vi "Main_量測.vi"(10 "連線測試":bool) -> ()   [LabVIEW 2015]
uses:
  Setting/0.Control/Setting_Control_Pattern Paremeter.ctl
  <vilib>/vision/Measure.llb/Edge Polarity.ctl
  Setting/0.Control/Setting_Control_Line Paremeter.ctl
  <vilib>/userdefined/High Color/IMAQdx.ctl
  <vilib>/Utility/miscctls.llb/LVPointTypeDef.ctl
  Function/1.0 IO/Control/Main_IO #.ctl
  <vilib>/vision/NI_Vision_Development_Module.lvlib
panel:
  out "狀態： 2":T1
  out "群組： 2":T2
  out "狀態：":string
  out "群組：":string
  out "帳號：":string
  in  "刀數 2":u16
  in  "功率右 2":i32=70 max=80
  in  "掃描速率(刀速)右 2":i32=220 max=2000 format="%0.0f"
  in  "角度(右) 3":dbl min=0.0 max=360.0
  in  "功率左 2":i32=70 max=80
  in  "掃描速率(刀速) 左 2":i32=220 max=2000 format="%0.0f"
  in  "角度(左) 3":dbl min=0.0 max=360.0
  in  "刀數":u16
  in  "功率右":i32=70 max=80
  in  "掃描速率(刀速)右":i32=220 max=2000 format="%0.0f"
  in  "角度(右)":dbl min=0.0 max=360.0
  in  "功率左":i32=70 max=80
  in  "掃描速率(刀速) 左":i32=220 max=2000 format="%0.0f"
  in  "角度(左)":dbl min=0.0 max=360.0
  in  "儲存圖片":bool
  in  "Tab Control":enum32{"影像1", "影像2"}(tab)
  out "Image1":T3(plugin-control)
  in  "pixel轉mm(左)":dbl
  out "總值左out":dbl
  in  "左邊線段":enum16{"加", "減"}(ring)
  in  "左進點":dbl
  in  "影像1左確認":bool
  in  "影像1右確認":bool
  out "總值右out":dbl
  in  "右邊線段":enum16{"加", "減"}(ring)
  in  "右進點":dbl
  out "Image 2":T3(plugin-control)
  in  "pixel轉mm(右)":dbl
  in  "影像2左確認":bool
  out "總值左out 2":dbl
  in  "左進點 2":dbl
  in  "左邊線段 2":enum16{"加", "減"}(ring)
  out "總值右out 2":dbl
  in  "右邊線段 2":enum16{"加", "減"}(ring)
  in  "右進點 2":dbl
  in  "影像2右確認":bool
  in  "代刚":bool
  in  "Enum":enum16{"オ", "右"}(ring)
  in  "代刚":bool
  out "Patttern_R":T3(plugin-control)
  out "Patttern_L":T3(plugin-control)
  out "連線測試 Action":T4
  # "不要的，試機時要拿掉"
  # "mm"
  # "mm"
  # "mm"
  # "mm"
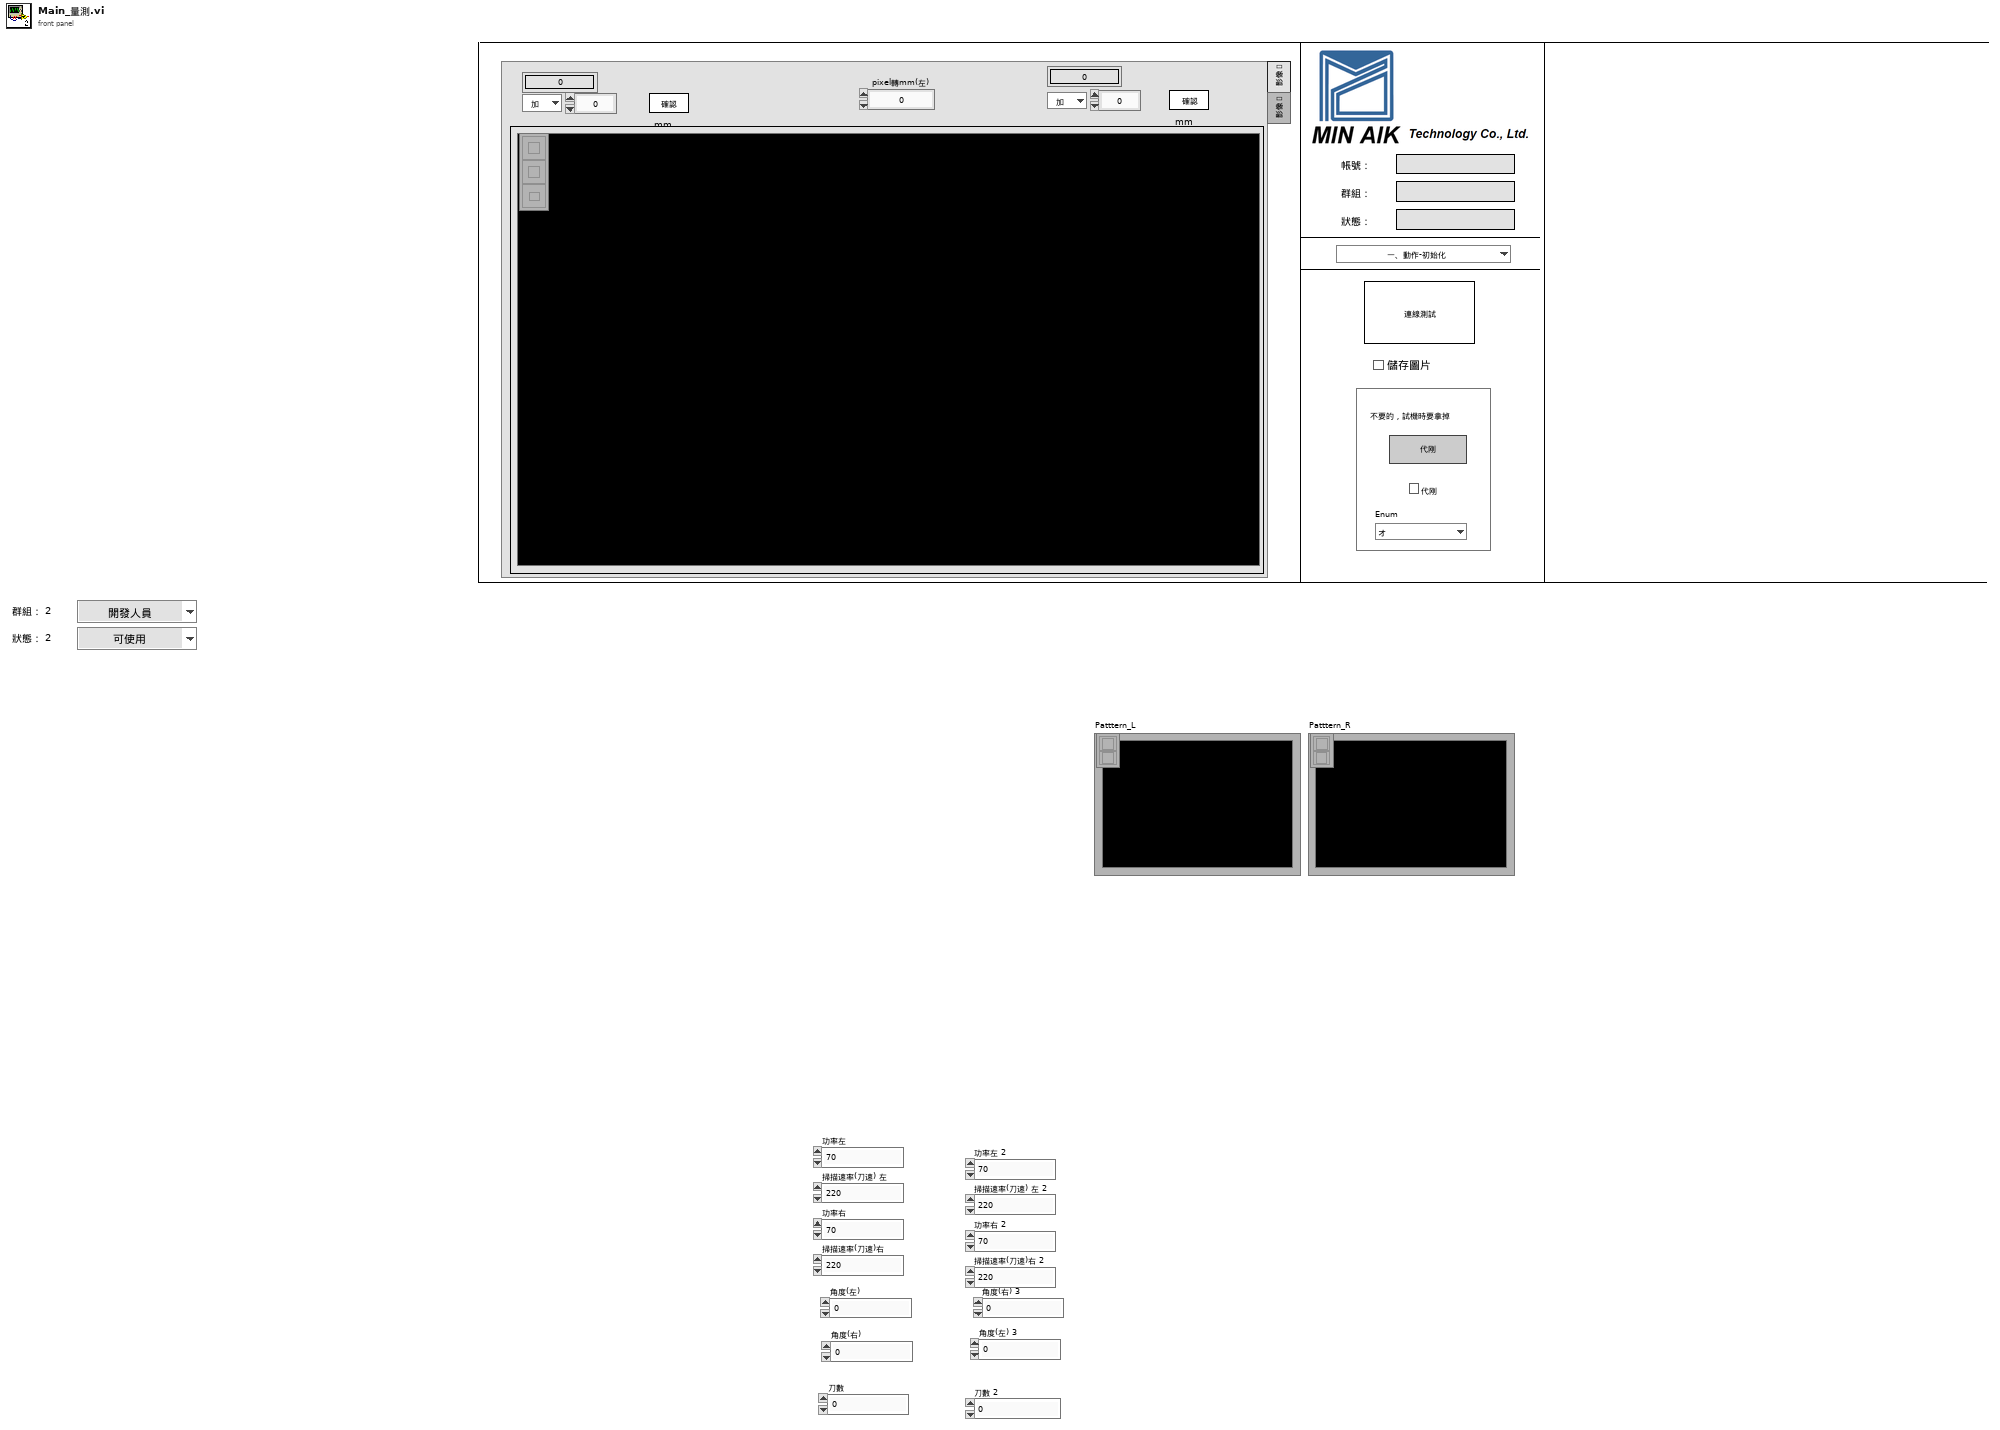
[diagram p1: front panel]
types:
  T1 = typedef "Control_User Accounts_Status.ctl" = enum16{"可使用", "不可使用"}
  T2 = typedef "Control_User account_Permissions.ctl" = enum16{"開發人員", "管理者", "工程師", "作業員"}
  T3 = typedef "IMAQ Image.ctl" = refnum<image>
  T4 = typedef "連線測試_Control_Main Action.ctl" = enum16{"一、動作-初始化", "二、動作-連線測試", "三、動作-離開", "1.0 功能-IO控制", "       1.1 IO-初始化", "       1.2 Set Point(EOT On)第一拍照", "       1.3Set Point(EOT Off)第一拍照", "       1.4Get Point(SOT)第一拍照", "       1.5Set Point(EOT On)第二拍照", "       1.6Set Point(EOT Off)第二拍照", "       1.7Get Point(SOT)第二拍照", "       1.8Set Point(EOT On)第一雷射", "       1.9Set Point(EOT Off)第一雷射", "       1.10Get Point(SOT)第一雷射", "       1.11Set Point(EOT On)第二雷射", "       1.12Set Point(EOT Off)第二雷射", "       1.13Get Point(SOT)第二雷射", "2.0功能-相機控制", "       2.1相機-初始化", "       2.2相機-取像1", "       2.2相機-取像2", "       2.3相機-關閉", "3.0功能-影像控制", "       3.1影像-初始化", "       3.2影像-更新影像", "       3.3影像-儲存影像1", "       3.3影像-儲存影像2", "4.0功能-檢測", "       4.1檢測-初始化", "      4.2浪代-浪代1", "      4.2浪代-浪代2", "      4.3檢測-量測1", "      4.3檢測-量測2", "5.0功能-雷射控制", "      5.1雷射-初始化", "      5.2雷射-寫入數值1", "      5.2雷射-寫入數值2", "      5.3雷射-寫入刀數", "      5.4雷射-讀出數值", "      5.5雷射-切換", "      5.6雷射-雷射觸發", "      5.7雷射-關閉", "6.0功能-檔案", "       6.1檔案-初始化", "       6.2檔案-儲存檔案", "       6.3檔案-開啟檔案(setting)", "       6.3檔案-開啟檔案(點檢)", "       6.3檔案-開啟檔案(近點)", "       6.4檔案-匯入檔案(近點)", "       6.4檔案-開啟檔案(雷射)", "7.0 錯誤", "8.0等待", "       8.1等待(計算時間)", "9.0離開", "10.0功能-機台驗證", "      10.1機台驗證-初始化", "      10.2機台驗證-檢測", "11.0對話視窗"}
  T5 = typedef "Control_Main_All Data.ctl" = enum16{"Initialize", "Set Data", "Get Data"}
  T6 = typedef "LVPointTypeDef.ctl" = cluster{"Horizontal":i16, "Vertical":i16}
  T7 = typedef "Control_User account_Data.ctl" = cluster{"帳號 :":string, "權限等級：":T2, "建立時間：":string, "修改時間：":string, "到期時間：":string, "狀態：":T1, "期限：":T8, "密碼：":string}
  T8 = typedef "Control_User account_Date.ctl" = enum16{"零天", "一天", "七天", "一個月", "一年", "三年"}
  T9 = enum8{"Enabled", "Disabled", "Disabled and Grayed Out"}
  T10 = typedef "IMAQdx.ctl" = refnum<k21>
  T11 = enum16{"Initialize", "Set Point", "Set Port", "Read Point", "Read Port", "Close", "Idle"}
  T12 = typedef "Main_IO #.ctl" = cluster{"CardID":u8, "Point#":u8, "Point Status":bool, "Port":u8, "Port Status":bool[]}
  T13 = typedef "action_camera.ctl" = enum16{"初始化", "取像", "匯入影像", "結束"}
  T14 = typedef "Image action.ctl" = enum16{"初始化", "創造記憶體", "寫入圖片", "讀取圖片", "刪除圖片", "等待"}
  T15 = cluster{"Brightness":sgl, "Contrast":sgl, "Gamma":sgl}
  T16 = typedef "Action_Data.ctl" = enum16{"Initialize", "Get Data", "Set Data", "Delete Data", "Idle"}
  T17 = typedef "Setting_Control_Line Paremeter.ctl" = cluster{"Search Direction":u32, "Edge Polarity":T18, "Kernel Size":u32, "Width":u32, "Minimum Edge Strength":sgl}
  T18 = typedef "Edge Polarity.ctl" = u32
  T19 = cluster{"邊參數R":T17, "ROI":cluster{"Global Rectangle":i32[], "Contours":cluster{"Contour Type":u32, "ROI Type":u32, "Points":i32[]}[]}}
  T20 = cluster{"邊參數L":T17, "ROI":cluster{"Global Rectangle":i32[], "Contours":cluster{"Contour Type":u32, "ROI Type":u32, "Points":i32[]}[]}}
  T21 = typedef "Setting_Control_Pattern Paremeter.ctl" = cluster{"方法":u16, "分數":sgl, "起始角度":sgl, "結束角度":sgl}
  T22 = typedef "IMAQ Coordinate System" = cluster{"Reference System":cluster{"Origin":cluster{"X":sgl, "Y":sgl}, "Angle (deg)":sgl, "Axis Reference":u32}, "Measurement System":cluster{"Origin":cluster{"X":sgl, "Y":sgl}, "Angle (deg)":sgl, "Axis Reference":u32}}
  T23 = cluster{"ROI":cluster{"Global Rectangle":i32[], "Contours":cluster{"Contour Type":u32, "ROI Type":u32, "Points":i32[]}[]}, "樣本比對參數R":T21, "Coordinate System Out":T22}
  T24 = cluster{"樣本比對參數L":T21, "ROI":cluster{"Global Rectangle":i32[], "Contours":cluster{"Contour Type":u32, "ROI Type":u32, "Points":i32[]}[]}, "Coordinate System Out":T22}
  T25 = cluster{"ROI":cluster{"Global Rectangle":i32[], "Contours":cluster{"Contour Type":u32, "ROI Type":u32, "Points":i32[]}[]}, "圓心 (Pixels)":cluster{"X":sgl, "Y":sgl}}
  T26 = cluster{"點1 (Pixels)":cluster{"X":sgl, "Y":sgl}, "點2 (Pixels)":cluster{"X":sgl, "Y":sgl}, "Angle (Pixel)":dbl}
  T27 = enum16{"RS232_Init ", "雷射準備訊號", "雷射觸發", "RS232_Close", "寫入雷射XY座標值與角度", "請求程式編號prog所有資訊", "開起導向光", "關閉導向光", "運行切換"}
  T28 = cluster{cluster{"掃描速度":i32, "功率":i32, "切割刀數":i32, "角度":dbl}, cluster{"掃描速度2":i32, "功率2":i32, "切割刀數2":i32, "角度2":dbl}, cluster{"掃描速度3":i32, "功率3":i32, "切割刀數3":i32, "角度3":dbl}, cluster{"掃描速度4":i32, "功率4":i32, "切割刀數4":i32, "角度4":dbl}, cluster{"掃描速度5":i32, "功率5":i32, "切割刀數5":i32}}
  T29 = cluster{"左X分量":dbl, "左Y分量":dbl, "右X分量":dbl, "右Y分量":dbl, "pixel轉mm(左)":dbl, "offect總值 out":cluster{"總值左out":dbl, "總值右out ":dbl}}
  T30 = cluster{"左X分量":dbl, "左Y分量":dbl, "右X分量":dbl, "右Y分量":dbl, "pixel轉mm(右)":dbl, "offect總值 out":cluster{"總值左out":dbl, "總值右out ":dbl}}
  T31 = cluster{cluster{"掃描速度":i32, "功率":i32, "切割刀數":i32, "角度":dbl}, cluster{"掃描速度2":i32, "功率2":i32, "切割刀數":i32, "角度2":dbl}, cluster{"掃描速度3":i32, "功率3":i32, "切割刀數3":i32, "角度3":dbl}, cluster{"掃描速度4":i32, "功率4":i32, "切割刀數3":i32, "角度4":dbl}, cluster{"掃描速率(刀速) ":u16, "功率":u8, "刀數":u32}}
  T32 = enum16{"RS232_Init ", "雷射準備訊號", "雷射觸發", "RS232_Close", "寫入雷射XY座標值與角度", "請求程式編號prog所有資訊", "開起導向光", "關閉導向光"}
  T33 = cluster{"Distances左水平(mm)":dbl, "Distance左垂直(mm)":dbl, "Distances右水平(mm)":dbl, "Distance右垂直(mm)":dbl, "pixel轉mm(右)":dbl, "總值 out":cluster{"總值左out":dbl, "總值右out ":dbl}}
  T34 = cluster{"Distances左水平(mm)":dbl, "Distance左垂直(mm)":dbl, "Distances右水平(mm)":dbl, "Distance右垂直(mm)":dbl, "pixel轉mm(左)":dbl, "總值 out":cluster{"總值左out":dbl, "總值右out ":dbl}}
  T35 = typedef "Image Type" = u32
  T36 = cluster{"Global Rectangle":i32[], "Contours":cluster{"Contour Type":u32, "ROI Type":u32, "Points":i32[]}[]}
  T37 = cluster{"掃描速度":i32, "功率":i32, "切割刀數":i32, "角度":dbl}
  T38 = cluster{"掃描速度2":i32, "功率2":i32, "切割刀數2":i32, "角度2":dbl}
  T39 = cluster{"掃描速度3":i32, "功率3":i32, "切割刀數3":i32, "角度3":dbl}
  T40 = cluster{"掃描速度4":i32, "功率4":i32, "切割刀數4":i32, "角度4":dbl}
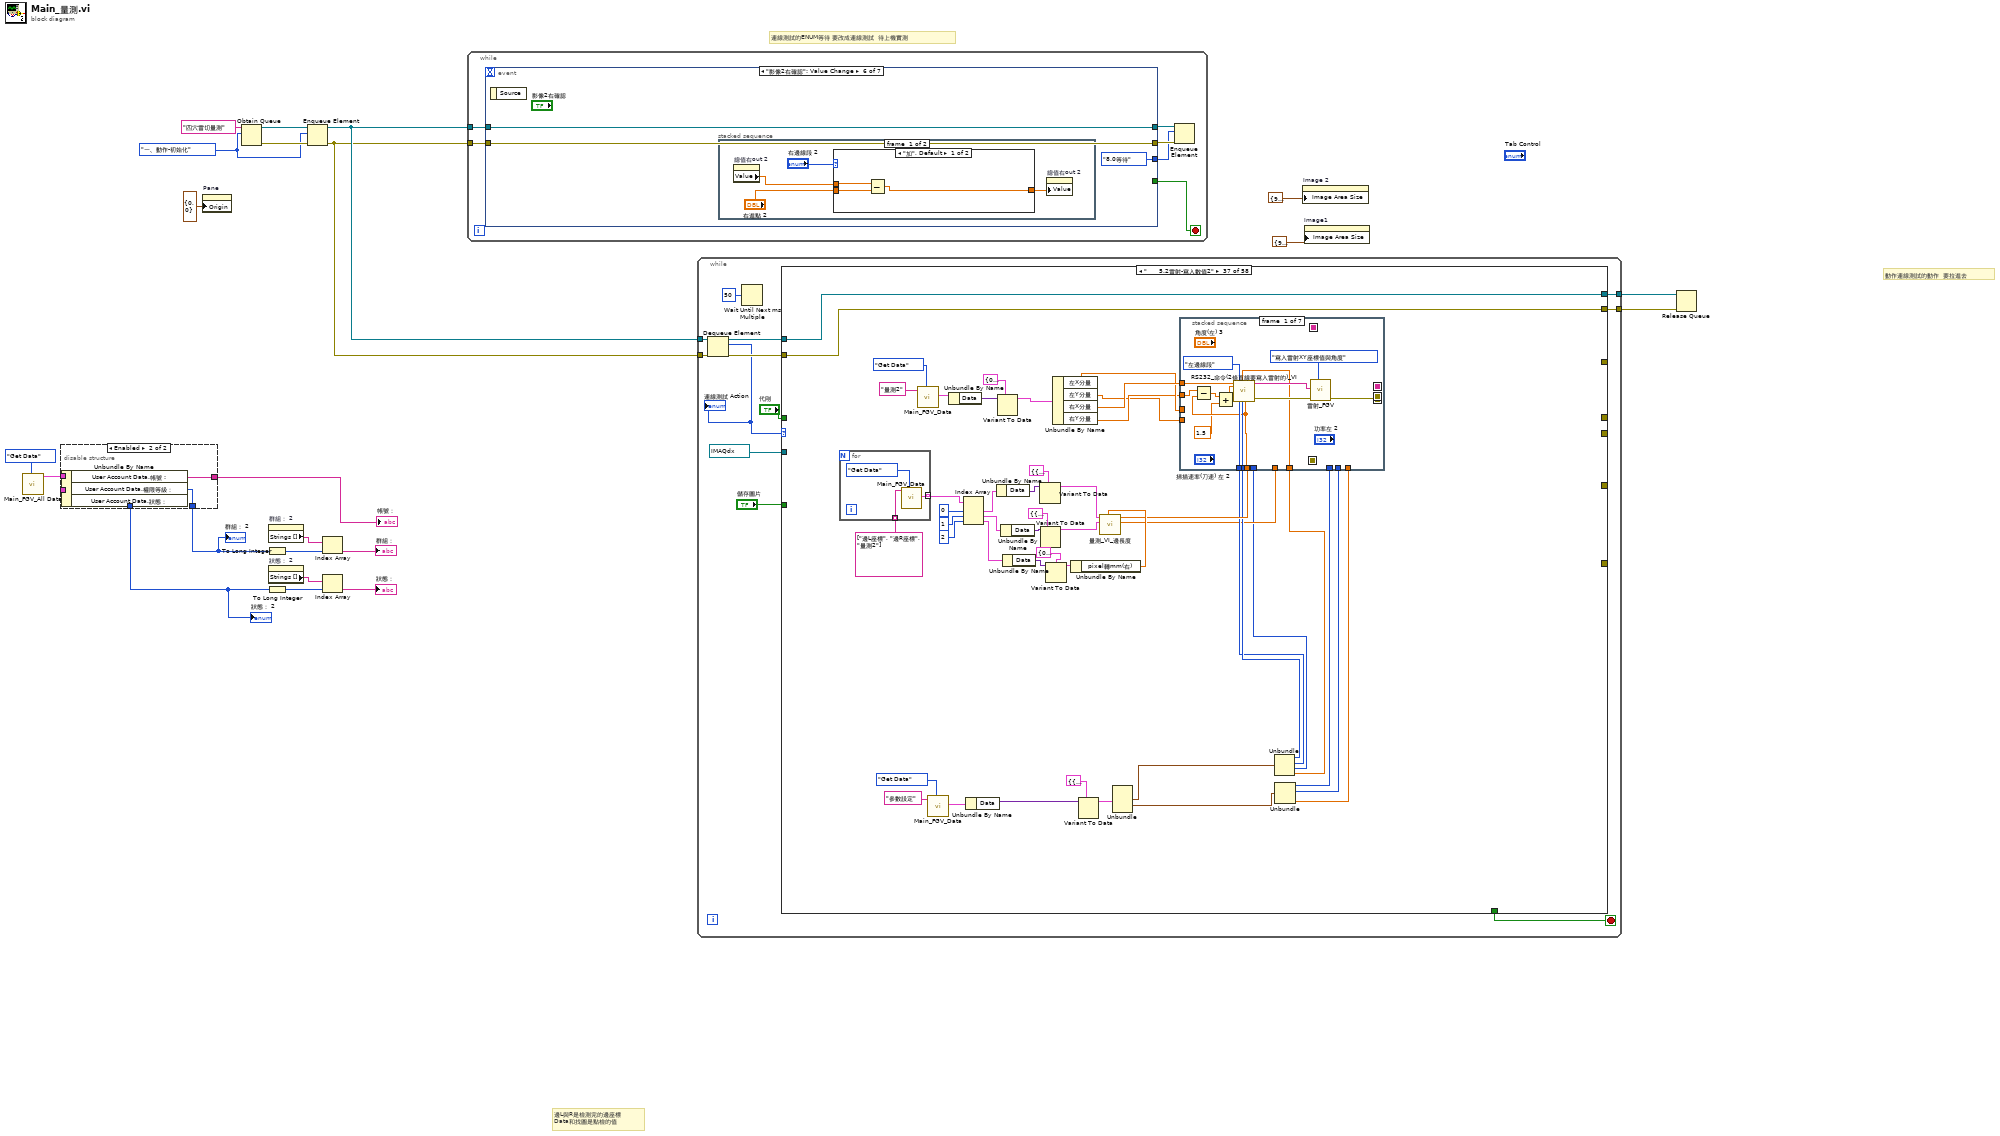
[diagram p0: block diagram]
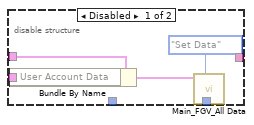
[diagram p2: hidden frame]
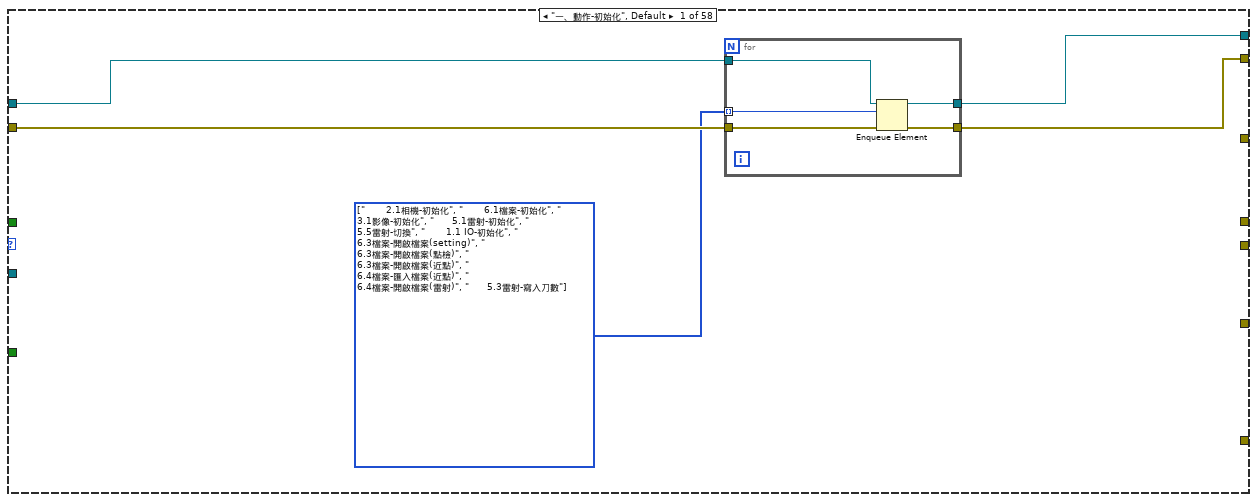
[diagram p3: hidden frame]
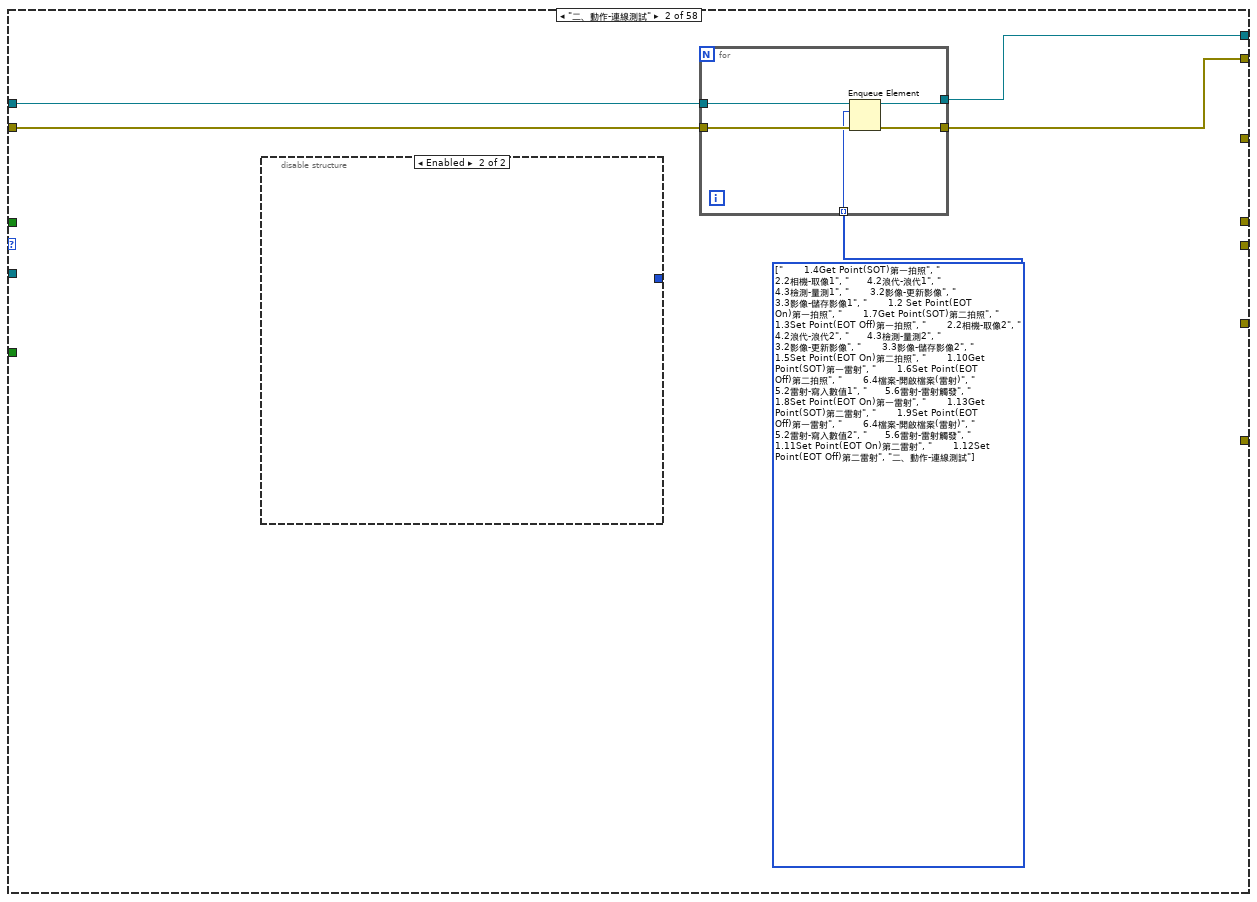
[diagram p4: hidden frame]
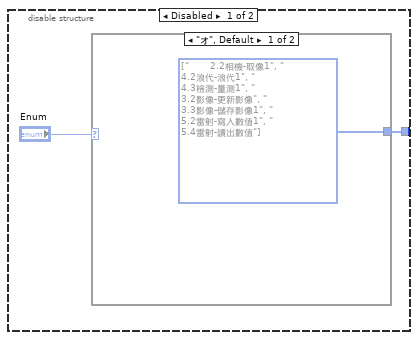
[diagram p5: hidden frame]
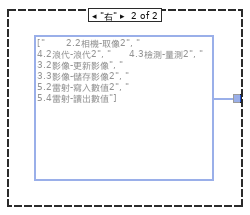
[diagram p6: hidden frame]
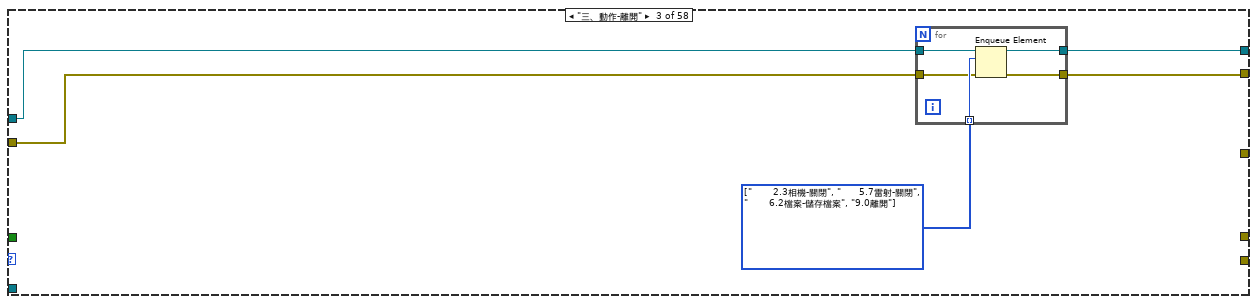
[diagram p7: hidden frame]
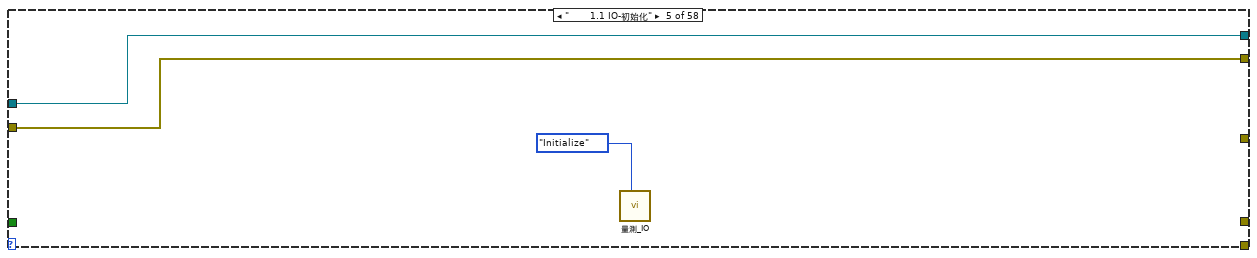
[diagram p9: hidden frame]
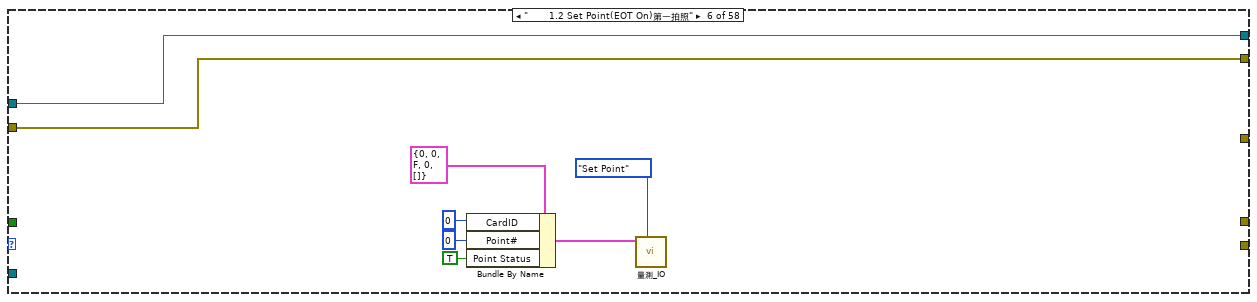
[diagram p10: hidden frame]
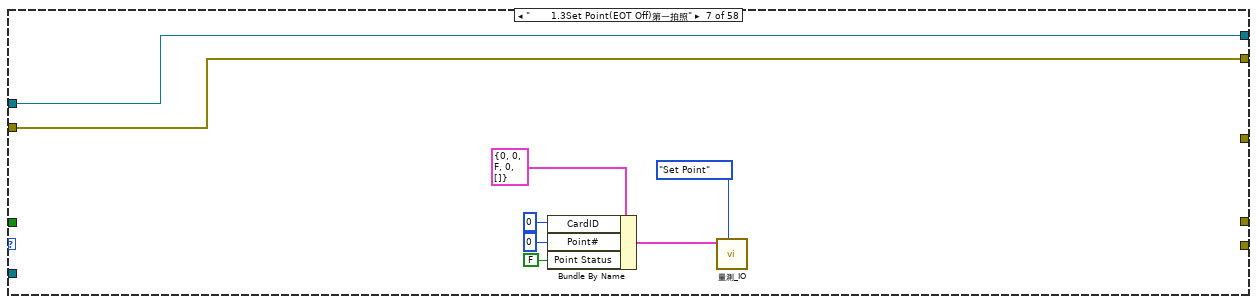
[diagram p11: hidden frame]
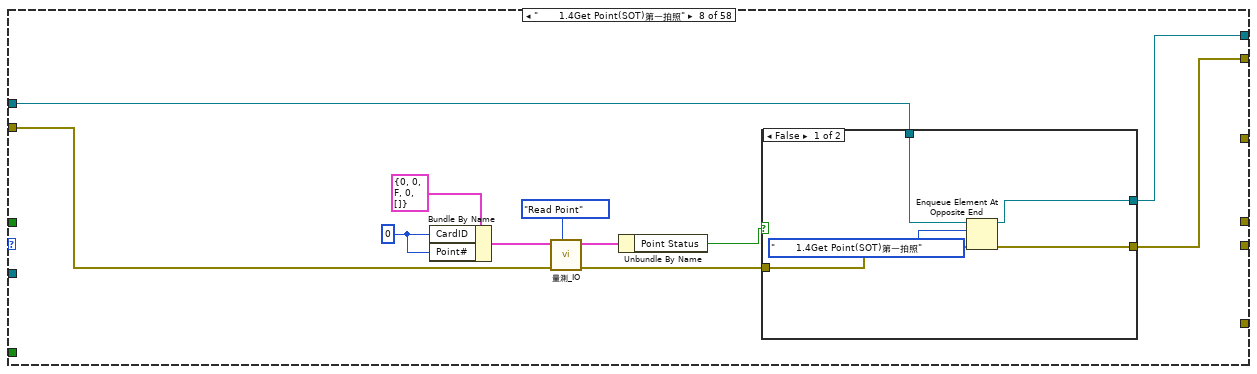
[diagram p12: hidden frame]
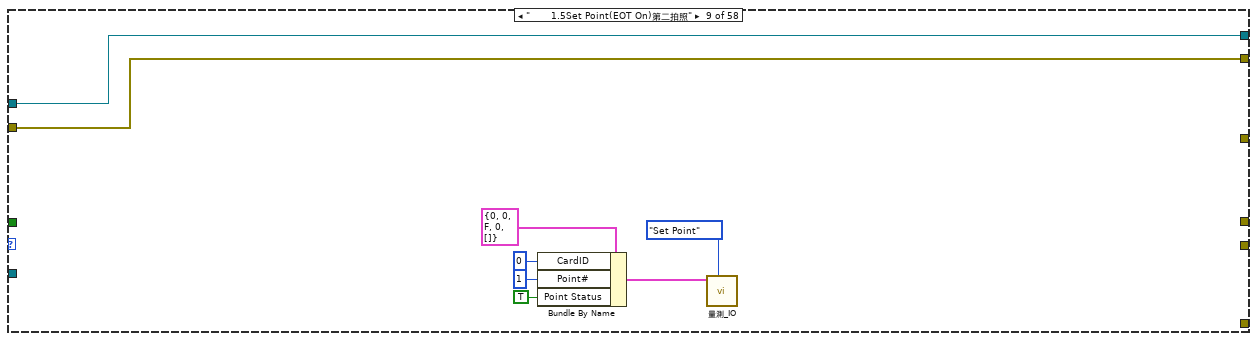
[diagram p14: hidden frame]
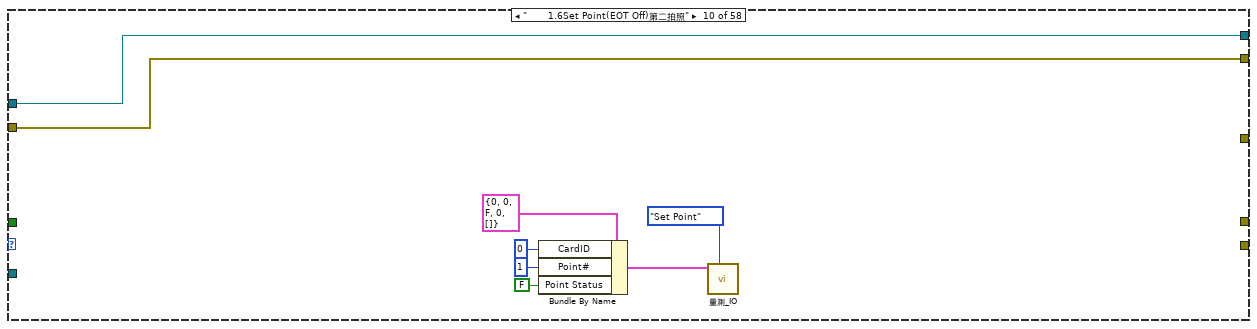
[diagram p15: hidden frame]
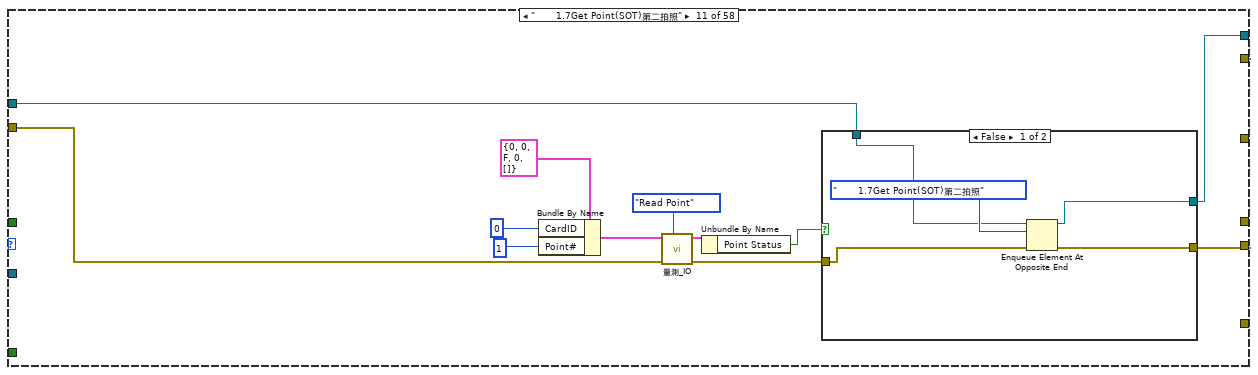
[diagram p16: hidden frame]
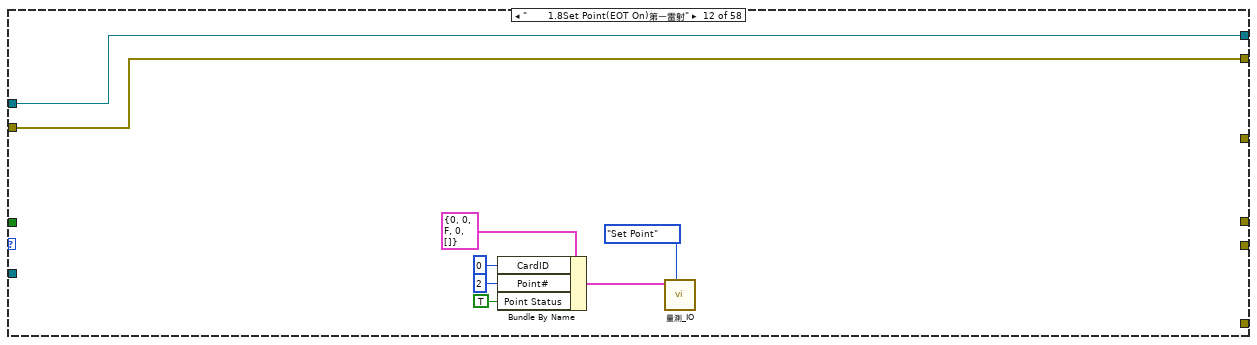
[diagram p18: hidden frame]
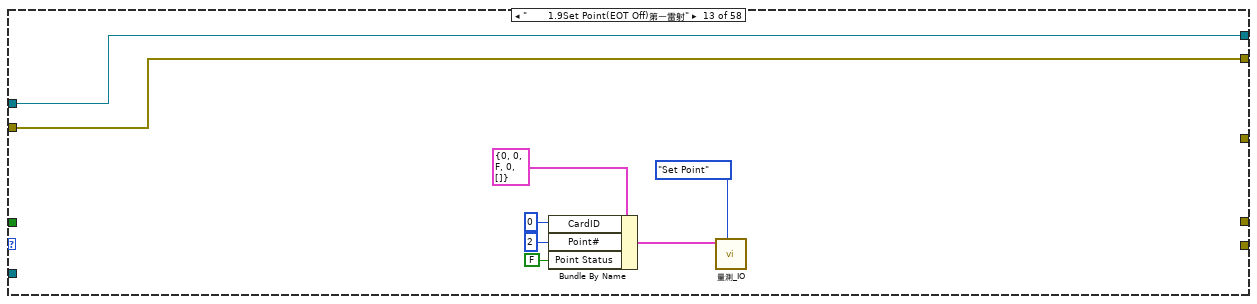
[diagram p19: hidden frame]
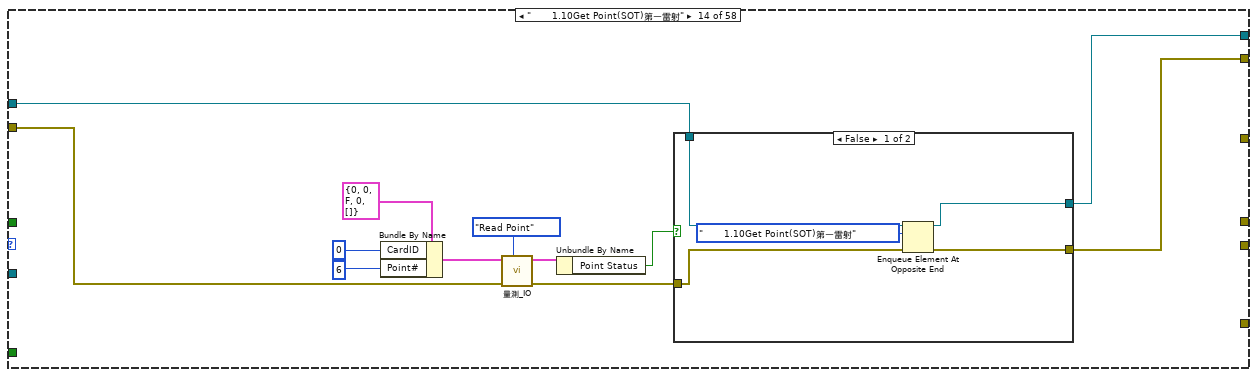
[diagram p20: hidden frame]
diagram:
  w19 = 連線測試_Control_Main_Action."一、動作-初始化" ("連線測試 Action")
  # "邊L與R是檢測完的邊座標\nData和找圓是點檢的值"
  # "動作連線測試的動作  要拉進去"
  # "連線測試的ENUM等待 要改成連線測試  待上機實測"
  n1 = call "Main_FGV_All Data.vi"("Data_Action"=Control_Main_All_Data."Get Data") -> ("All Data Out"=w10:cluster{"User Account Data":T7})  [unwired: 9 in, 1 out]
  n2 = disable-structure shown="Enabled" {
    disable-tunnel: w10 -> [w26 w30]
    disable-tunnel: _ -> [w23 _]
    disable-tunnel: [_ w29] -> w3
    disable-tunnel: [_ w28] -> w2
    disable-tunnel: [_ w27] -> w1
    frame Disabled {
      n3 = Bundle By Name(cluster=w26, "User Account Data"=w23) -> (w24:cluster{"User Account Data":T7})
      n4 = call "Main_FGV_All Data.vi"("Data_Action"=Control_Main_All_Data."Set Data", "All Data In"=w24) -> ()  [unwired: 8 in, 2 out]
    }
    frame Enabled {
      n5 = Unbundle By Name(w30) -> ("User Account Data.帳號 :"=w29:string, "User Account Data.權限等級："=w28:T2, "User Account Data.狀態："=w27:T1)
    }
  }
  "帳號：" <- w3
  "群組： 2" <- w2
  "狀態： 2" <- w1
  n6 = property on="Pane" class="Pane"("Origin"=T6 {"Horizontal"=0, "Vertical"=0}) -> ()  [unwired: 2 in, 2 out]
  n7 = Obtain Queue(name (unnamed)="四穴雷切量測", element data type=w19) -> (queue out=w21:refnum<queue>, error out=w20:errorcluster)  [unwired: 3 in, 1 out]
  n8 = To Long Integer(number=w2) -> (32bit integer=w7:i32)
  n9 = To Long Integer(number=w1) -> (32bit integer=w6:i32)
  n10 = property on="群組： 2" class="Enum (strict)"() -> ("Strings []"=w9:string[])  [unwired: 2 in, 2 out]
  n11 = property on="狀態： 2" class="Enum (strict)"() -> ("Strings []"=w8:string[])  [unwired: 2 in, 2 out]
  n12 = Enqueue Element(queue=w21, element=w19, error in (no error)=w20) -> (queue out=w18:refnum<queue>, error out=w12:errorcluster)  [unwired: 1 in, 1 out]
  n13 = Index Array(array=w9, index=w7) -> (element=→"群組：":string)
  n14 = Index Array(array=w8, index=w6) -> (element=→"狀態：":string)
  n15 = while {
    tunnel: w18 -> [w36]
    tunnel: w12 -> [w35]
    stop <- w31 stop-if-true
    n16 = event shown="[5] \"影像2右確認\": Value Change" {
      selector: _ -> [_ _ _ _ _ _ _]
      dyn-events: _ -> [_ _ _ _ _ _ _]
      timeout: _ -> [_ _ _ _ _ _ _]
      tunnel: [w38 w43 w60 w73 w88 w102 w116] -> w34
      tunnel: w36 -> [w38 w45 w60 w73 w88 w102 w116]
      tunnel: w35 -> [w37 w44 w59 w72 w87 w101 w115]
      tunnel: [w37 w42 w59 w72 w87 w101 w115] -> w33
      tunnel: [_ w41 連線測試_Control_Main_Action."8.0等待" ("連線測試 Action") 連線測試_Control_Main_Action."8.0等待" ("連線測試 Action") 連線測試_Control_Main_Action."8.0等待" ("連線測試 Action") 連線測試_Control_Main_Action."8.0等待" ("連線測試 Action") 連線測試_Control_Main_Action."二、動作-連線測試" ("連線測試 Action")] -> w32
      tunnel: [_ w40 _ _ _ _ _] -> w31
      event Timeout {
        n17 = event-data() -> ()  [unwired: 1 in, 1 out]
      }
      event "連線測試": Value Change {
        n18 = event-data() -> ()  [unwired: 1 in, 1 out]
        n19 = case shown="True" "連線測試" {
          tunnel: w45 -> [w49 w54]
          tunnel: w44 -> [w48 w53]
          tunnel: [w46 w54] -> w43
          tunnel: [w47 w53] -> w42
          tunnel: [連線測試_Control_Main_Action."三、動作-離開" ("連線測試 Action") 連線測試_Control_Main_Action."二、動作-連線測試" ("連線測試 Action")] -> w41
          tunnel: [TRUE _] -> w40
          frame False {
            n20 = Flush Queue(queue=w49, error in (no error)=w48) -> (queue out=w46:refnum<queue>, error out=w47:errorcluster)  [unwired: 1 out]
          }
          frame True {
            n21 = flat-sequence {
              frame #0 {
                n22 = property on="連線測試" class="Bool (strict)"("DisabledEnum"=T9."Disabled and Grayed Out" ("Disabled")) -> ()  [unwired: 2 in, 2 out]
              }
              frame #1 {
                n23 = Wait (ms)(milliseconds to wait=u32 1000) -> ()  [unwired: 1 out]
              }
              frame #2 {
                n24 = property on="連線測試" class="Bool (strict)"("DisabledEnum"=T9."Enabled" ("Disabled")) -> ()  [unwired: 2 in, 2 out]
              }
            }
          }
        }
      }
      event "影像1左確認": Value Change {
        n25 = event-data() -> ()  [unwired: 1 in, 1 out]
        n26 = stacked-sequence {
          frame #0 {
            n27 = property on="總值左out" class="DigNum (strict)"() -> ("Value"=w64:dbl)  [unwired: 2 in, 2 out]
            n28 = case shown="\"加\", Default" "左邊線段" {
              tunnel: w64 -> [w67 w70]
              tunnel: [w66 w68] -> w63
              tunnel: "左進點" -> [w65 w69]
              frame "加", Default {
                n29 = Add(x=w67, y=w65) -> (x+y=w66:dbl)
              }
              frame "減" {
                n30 = Subtract(x=w70, y=w69) -> (x-y=w68:dbl)
              }
            }
            n31 = property on="總值左out" class="DigNum (strict)"("Value"=w63) -> ()  [unwired: 2 in, 2 out]
          }
          frame #1 {
            n32 = property on="左進點" class="DigNum (strict)"("Value"=0.0) -> ()  [unwired: 2 in, 2 out]
          }
        }
      }
      event "影像1右確認": Value Change {
        n33 = event-data() -> ()  [unwired: 1 in, 1 out]
        n34 = stacked-sequence {
          frame #0 {
            n35 = property on="總值右out" class="DigNum (strict)"() -> ("Value"=w77:dbl)  [unwired: 2 in, 2 out]
            n36 = case shown="\"加\", Default" "右邊線段" {
              tunnel: w77 -> [w81 w84]
              tunnel: "右進點" -> [w80 w83]
              tunnel: [w79 w82] -> w75
              frame "加", Default {
                n37 = Subtract(x=w81, y=w80) -> (x-y=w79:dbl)
              }
              frame "減" {
                n38 = Add(x=w84, y=w83) -> (x+y=w82:dbl)
              }
            }
            n39 = property on="總值右out" class="DigNum (strict)"("Value"=w75) -> ()  [unwired: 2 in, 2 out]
          }
          frame #1 {
            n40 = property on="右進點" class="DigNum (strict)"("Value"=0.0) -> ()  [unwired: 2 in, 2 out]
          }
        }
      }
      event "影像2左確認": Value Change {
        n41 = event-data() -> ()  [unwired: 1 in, 1 out]
        n42 = stacked-sequence {
          frame #0 {
            n43 = property on="總值左out 2" class="DigNum (strict)"() -> ("Value"=w90:dbl)  [unwired: 2 in, 2 out]
            n44 = case shown="\"加\", Default" "左邊線段 2" {
              tunnel: "左進點 2" -> [w95 w98]
              tunnel: w90 -> [w94 w97]
              tunnel: [w93 w96] -> w89
              frame "加", Default {
                n45 = Add(x=w94, y=w95) -> (x+y=w93:dbl)
              }
              frame "減" {
                n46 = Subtract(x=w97, y=w98) -> (x-y=w96:dbl)
              }
            }
            n47 = property on="總值左out 2" class="DigNum (strict)"("Value"=w89) -> ()  [unwired: 2 in, 2 out]
          }
          frame #1 {
            n48 = property on="左進點 2" class="DigNum (strict)"("Value"=0.0 ("左進點 2")) -> ()  [unwired: 2 in, 2 out]
          }
        }
      }
      event "影像2右確認": Value Change {
        n49 = event-data() -> ()  [unwired: 1 in, 1 out]
        n50 = stacked-sequence {
          frame #0 {
            n51 = property on="總值右out 2" class="DigNum (strict)"() -> ("Value"=w104:dbl)  [unwired: 2 in, 2 out]
            n52 = case shown="\"加\", Default" "右邊線段 2" {
              tunnel: "右進點 2" -> [w108 w112]
              tunnel: w104 -> [w109 w111]
              tunnel: [w107 w110] -> w103
              frame "加", Default {
                n53 = Subtract(x=w109, y=w108) -> (x-y=w107:dbl)
              }
              frame "減" {
                n54 = Add(x=w111, y=w112) -> (x+y=w110:dbl)
              }
            }
            n55 = property on="總值右out 2" class="DigNum (strict)"("Value"=w103) -> ()  [unwired: 2 in, 2 out]
          }
          frame #1 {
            n56 = property on="右進點 2" class="DigNum (strict)"("Value"=0.0) -> ()  [unwired: 2 in, 2 out]
          }
        }
      }
      event "代刚": Value Change {
        n57 = event-data() -> ()  [unwired: 1 in, 1 out]
      }
    }
    n58 = Enqueue Element(queue=w34, element=w32, error in (no error)=w33) -> ()  [unwired: 1 in, 3 out]
  }
  n59 = while {
    tunnel: w18 -> [w128]
    tunnel: w12 -> [w127]
    tunnel: [w124] -> w17
    tunnel: [w123] -> w16
    stop <- w122 stop-if-true
    n60 = Dequeue Element(queue=w128, error in (no error)=w127) -> (queue out=w126:refnum<queue>, element=w121:T4, error out=w125:errorcluster)  [unwired: 1 in, 1 out]
    "連線測試 Action" <- w121
    n61 = Wait Until Next ms Multiple(millisecond multiple=u32 50) -> ()  [unwired: 1 out]
    n62 = case shown="\"      5.2雷射-寫入數值2\"" w121 {
      tunnel: w126 -> [w133 w143 w154 w164 w167 w175 w183 w188 w209 w217 w223 w244 w252 w258 w280 w288 w294 w309 w313 w316 w336 w355 w357 w363 w395 w412 w432 w449 w451 w513 w578 w625 w672 w677 w682 w729 w834 w906 w923 w925 w931 w947 w949 w952 w957 w990 w1009 w1022 w1049 w1055 w1060 w1062 w1064 w1068 w1071 w1073 w1075 w1077]
      tunnel: w125 -> [w132 w142 w153 w163 w166 w174 w182 w187 w208 w216 w222 w243 w251 w257 w279 w287 w293 w308 w312 w315 w335 w354 w356 w362 w394 w413 w431 w448 w450 w512 w577 w624 w671 w676 w681 w728 w833 w905 w922 w924 w930 w946 w948 w951 w956 w989 w1008 w1021 w1048 w1054 w1059 w1061 w1063 w1067 w1070 w1072 w1074 w1076]
      tunnel: [w131 w141 w157 w164 w167 w175 w183 w186 w209 w217 w220 w244 w252 w255 w280 w288 w291 w309 w313 w316 w336 w355 w357 w363 w395 w411 w430 w449 w451 w513 w578 w625 w672 w677 w682 w729 w834 w906 w923 w925 w931 w947 w949 w952 w957 w988 w1009 w1022 w1049 w1055 w1060 w1062 w1064 w1065 w1071 w1073 w1075 w1077] -> w124
      tunnel: [w130 w140 w156 w163 w166 w174 w182 w185 w208 w216 w219 w243 w251 w254 w279 w287 w290 w308 w312 w315 w335 w354 w356 w362 w394 w410 w429 w448 w450 w512 w577 w624 w671 w676 w681 w728 w833 w905 w922 w924 w930 w946 w948 w951 w956 w987 w1008 w1021 w1048 w1054 w1059 w1061 w1063 w1066 w1070 w1072 w1074 w1076] -> w123
      tunnel: [_ _ _ _ _ _ _ _ _ _ _ _ _ _ _ _ _ _ _ _ _ _ _ _ _ _ _ _ _ _ _ _ _ _ _ _ _ _ _ _ _ _ _ _ _ _ _ _ _ _ _ _ _ TRUE _ _ _ _] -> w122
      tunnel: T10 "cam0" ("Session In") -> [_ _ _ _ _ _ _ _ _ _ _ _ _ _ _ _ _ _ w310 w317 w333 w352 _ _ _ _ _ _ _ _ _ _ _ _ _ _ _ _ _ _ _ _ _ _ _ _ _ _ _ _ _ _ _ _ _ _ _ _]
      tunnel: [_ _ _ _ _ _ _ _ _ _ _ _ _ _ _ _ _ _ _ _ _ _ _ _ _ _ _ _ _ _ _ _ _ _ _ _ _ _ _ _ _ _ _ _ _ w964 _ _ _ _ _ _ _ _ _ _ _ _] -> _
      tunnel: [_ _ _ _ _ _ _ _ _ _ _ _ _ _ _ _ _ _ _ _ _ _ _ _ _ _ _ _ _ _ _ _ _ _ _ _ _ _ _ _ _ _ _ _ _ w963 _ _ w1038 _ _ _ _ _ _ _ _ _] -> _
      tunnel: [_ _ _ _ _ _ _ _ _ _ _ _ _ _ _ _ _ _ _ _ _ _ _ _ _ _ _ _ _ _ _ _ _ _ _ _ _ _ _ _ _ _ _ _ _ w962 _ _ _ _ _ _ _ _ _ _ _ _] -> _
      tunnel: "代刚" -> [_ _ _ _ _ _ _ _ _ _ _ _ _ _ _ _ _ _ _ w314 w334 _ _ _ _ _ _ _ _ _ _ _ _ _ _ _ _ _ _ _ _ _ _ _ _ _ _ _ _ _ _ _ _ _ _ _ _ _]
      tunnel: "儲存圖片" -> [_ _ _ _ _ _ _ _ _ _ _ _ _ _ _ _ _ _ _ _ _ _ _ _ _ w414 w433 _ _ _ _ _ _ _ _ _ _ _ _ _ _ _ _ _ _ _ _ _ _ _ _ _ _ _ _ _ _ _]
      tunnel: [_ _ _ _ _ _ _ _ _ _ _ _ _ _ _ _ _ _ _ _ _ _ _ _ w372 _ _ _ _ _ _ _ _ _ _ _ _ _ _ _ _ _ _ _ _ _ _ _ _ _ _ _ _ _ _ _ _ _] -> _
      tunnel: [_ _ _ _ _ _ _ _ _ _ _ _ _ _ _ _ _ _ _ _ _ _ _ _ w368 _ _ _ _ _ _ _ _ _ _ _ _ _ _ _ _ _ _ _ _ _ _ _ _ _ _ _ _ _ _ _ _ _] -> _
      frame "一、動作-初始化", Default {
        w129 = T4[] [enum."       2.1相機-初始化", enum."       6.1檔案-初始化", enum."       3.1影像-初始化", enum."      5.1雷射-初始化", enum."      5.5雷射-切換", enum."       1.1 IO-初始化", enum."       6.3檔案-開啟檔案(setting)", enum."       6.3檔案-開啟檔案(點檢)", enum."       6.3檔案-開啟檔案(近點)", enum."       6.4檔案-匯入檔案(近點)", enum."       6.4檔案-開啟檔案(雷射)", enum."      5.3雷射-寫入刀數"] items=["一、動作-初始化", "二、動作-連線測試", "三、動作-離開", "1.0 功能-IO控制", "       1.1 IO-初始化", "       1.2 Set Point(EOT On)第一拍照", "       1.3Set Point(EOT Off)第一拍照", "       1.4Get Point(SOT)第一拍照", "       1.5Set Point(EOT On)第二拍照", "       1.6Set Point(EOT Off)第二拍照", "       1.7Get Point(SOT)第二拍照", "       1.8Set Point(EOT On)第一雷射", "       1.9Set Point(EOT Off)第一雷射", "       1.10Get Point(SOT)第一雷射", "       1.11Set Point(EOT On)第二雷射", "       1.12Set Point(EOT Off)第二雷射", "       1.13Get Point(SOT)第二雷射", "2.0功能-相機控制", "       2.1相機-初始化", "       2.2相機-取像1", "       2.2相機-取像2", "       2.3相機-關閉", "3.0功能-影像控制", "       3.1影像-初始化", "       3.2影像-更新影像", "       3.3影像-儲存影像1", "       3.3影像-儲存影像2", "4.0功能-檢測", "       4.1檢測-初始化", "      4.2浪代-浪代1", "      4.2浪代-浪代2", "      4.3檢測-量測1", "      4.3檢測-量測2", "5.0功能-雷射控制", "      5.1雷射-初始化", "      5.2雷射-寫入數值1", "      5.2雷射-寫入數值2", "      5.3雷射-寫入刀數", "      5.4雷射-讀出數值", "      5.5雷射-切換", "      5.6雷射-雷射觸發", "      5.7雷射-關閉", "6.0功能-檔案", "       6.1檔案-初始化", "       6.2檔案-儲存檔案", "       6.3檔案-開啟檔案(setting)", "       6.3檔案-開啟檔案(點檢)", "       6.3檔案-開啟檔案(近點)", "       6.4檔案-匯入檔案(近點)", "       6.4檔案-開啟檔案(雷射)", "7.0 錯誤", "8.0等待", "       8.1等待(計算時間)", "9.0離開", "10.0功能-機台驗證", "      10.1機台驗證-初始化", "      10.2機台驗證-檢測", "11.0對話視窗"]
        n63 = for {
          tunnel: w133 -> [w138]
          tunnel: w132 -> [w137]
          tunnel: [w136] -> w130
          tunnel: [w135] -> w131
          tunnel: w129 -> [w134] mode=indexing
          n64 = Enqueue Element(queue=w138, element=w134, error in (no error)=w137) -> (queue out=w135:refnum<queue>, error out=w136:errorcluster)  [unwired: 1 in, 1 out]
        }
      }
      frame "二、動作-連線測試" {
        w139 = T4[] [enum."       1.4Get Point(SOT)第一拍照", enum."       2.2相機-取像1", enum."      4.2浪代-浪代1", enum."      4.3檢測-量測1", enum."       3.2影像-更新影像", enum."       3.3影像-儲存影像1", enum."       1.2 Set Point(EOT On)第一拍照", enum."       1.7Get Point(SOT)第二拍照", enum."       1.3Set Point(EOT Off)第一拍照", enum."       2.2相機-取像2", enum."      4.2浪代-浪代2", enum."      4.3檢測-量測2", enum."       3.2影像-更新影像", enum."       3.3影像-儲存影像2", enum."       1.5Set Point(EOT On)第二拍照", enum."       1.10Get Point(SOT)第一雷射", enum."       1.6Set Point(EOT Off)第二拍照", enum."       6.4檔案-開啟檔案(雷射)", enum."      5.2雷射-寫入數值1", enum."      5.6雷射-雷射觸發", enum."       1.8Set Point(EOT On)第一雷射", enum."       1.13Get Point(SOT)第二雷射", enum."       1.9Set Point(EOT Off)第一雷射", enum."       6.4檔案-開啟檔案(雷射)", enum."      5.2雷射-寫入數值2", enum."      5.6雷射-雷射觸發", enum."       1.11Set Point(EOT On)第二雷射", enum."       1.12Set Point(EOT Off)第二雷射", enum."二、動作-連線測試"] items=["一、動作-初始化", "二、動作-連線測試", "三、動作-離開", "1.0 功能-IO控制", "       1.1 IO-初始化", "       1.2 Set Point(EOT On)第一拍照", "       1.3Set Point(EOT Off)第一拍照", "       1.4Get Point(SOT)第一拍照", "       1.5Set Point(EOT On)第二拍照", "       1.6Set Point(EOT Off)第二拍照", "       1.7Get Point(SOT)第二拍照", "       1.8Set Point(EOT On)第一雷射", "       1.9Set Point(EOT Off)第一雷射", "       1.10Get Point(SOT)第一雷射", "       1.11Set Point(EOT On)第二雷射", "       1.12Set Point(EOT Off)第二雷射", "       1.13Get Point(SOT)第二雷射", "2.0功能-相機控制", "       2.1相機-初始化", "       2.2相機-取像1", "       2.2相機-取像2", "       2.3相機-關閉", "3.0功能-影像控制", "       3.1影像-初始化", "       3.2影像-更新影像", "       3.3影像-儲存影像1", "       3.3影像-儲存影像2", "4.0功能-檢測", "       4.1檢測-初始化", "      4.2浪代-浪代1", "      4.2浪代-浪代2", "      4.3檢測-量測1", "      4.3檢測-量測2", "5.0功能-雷射控制", "      5.1雷射-初始化", "      5.2雷射-寫入數值1", "      5.2雷射-寫入數值2", "      5.3雷射-寫入刀數", "      5.4雷射-讀出數值", "      5.5雷射-切換", "      5.6雷射-雷射觸發", "      5.7雷射-關閉", "6.0功能-檔案", "       6.1檔案-初始化", "       6.2檔案-儲存檔案", "       6.3檔案-開啟檔案(setting)", "       6.3檔案-開啟檔案(點檢)", "       6.3檔案-開啟檔案(近點)", "       6.4檔案-匯入檔案(近點)", "       6.4檔案-開啟檔案(雷射)", "7.0 錯誤", "8.0等待", "       8.1等待(計算時間)", "9.0離開", "10.0功能-機台驗證", "      10.1機台驗證-初始化", "      10.2機台驗證-檢測", "11.0對話視窗"]
        n65 = disable-structure shown="Enabled" {
          disable-tunnel: [w145 _] -> _
          frame Disabled {
            n66 = case shown="\"オ\", Default" "Enum" {
              tunnel: [w146 w147] -> w145
              frame "オ", Default {
                w146 = T4[] [enum."       2.2相機-取像1", enum."      4.2浪代-浪代1", enum."      4.3檢測-量測1", enum."       3.2影像-更新影像", enum."       3.3影像-儲存影像1", enum."      5.2雷射-寫入數值1", enum."      5.4雷射-讀出數值"] items=["一、動作-初始化", "二、動作-連線測試", "三、動作-離開", "1.0 功能-IO控制", "       1.1 IO-初始化", "       1.2 Set Point(EOT On)第一拍照", "       1.3Set Point(EOT Off)第一拍照", "       1.4Get Point(SOT)第一拍照", "       1.5Set Point(EOT On)第二拍照", "       1.6Set Point(EOT Off)第二拍照", "       1.7Get Point(SOT)第二拍照", "       1.8Set Point(EOT On)第一雷射", "       1.9Set Point(EOT Off)第一雷射", "       1.10Get Point(SOT)第一雷射", "       1.11Set Point(EOT On)第二雷射", "       1.12Set Point(EOT Off)第二雷射", "       1.13Get Point(SOT)第二雷射", "2.0功能-相機控制", "       2.1相機-初始化", "       2.2相機-取像1", "       2.2相機-取像2", "       2.3相機-關閉", "3.0功能-影像控制", "       3.1影像-初始化", "       3.2影像-更新影像", "       3.3影像-儲存影像1", "       3.3影像-儲存影像2", "4.0功能-檢測", "       4.1檢測-初始化", "      4.2浪代-浪代1", "      4.2浪代-浪代2", "      4.3檢測-量測1", "      4.3檢測-量測2", "5.0功能-雷射控制", "      5.1雷射-初始化", "      5.2雷射-寫入數值1", "      5.2雷射-寫入數值2", "      5.3雷射-寫入刀數", "      5.4雷射-讀出數值", "      5.5雷射-切換", "      5.6雷射-雷射觸發", "      5.7雷射-關閉", "6.0功能-檔案", "       6.1檔案-初始化", "       6.2檔案-儲存檔案", "       6.3檔案-開啟檔案(setting)", "       6.3檔案-開啟檔案(點檢)", "       6.3檔案-開啟檔案(近點)", "       6.4檔案-匯入檔案(近點)", "       6.4檔案-開啟檔案(雷射)", "7.0 錯誤", "8.0等待", "       8.1等待(計算時間)", "9.0離開", "10.0功能-機台驗證", "      10.1機台驗證-初始化", "      10.2機台驗證-檢測", "11.0對話視窗"]
              }
              frame "右" {
                w147 = T4[] [enum."       2.2相機-取像2", enum."      4.2浪代-浪代2", enum."      4.3檢測-量測2", enum."       3.2影像-更新影像", enum."       3.3影像-儲存影像2", enum."      5.2雷射-寫入數值2", enum."      5.4雷射-讀出數值"] items=["一、動作-初始化", "二、動作-連線測試", "三、動作-離開", "1.0 功能-IO控制", "       1.1 IO-初始化", "       1.2 Set Point(EOT On)第一拍照", "       1.3Set Point(EOT Off)第一拍照", "       1.4Get Point(SOT)第一拍照", "       1.5Set Point(EOT On)第二拍照", "       1.6Set Point(EOT Off)第二拍照", "       1.7Get Point(SOT)第二拍照", "       1.8Set Point(EOT On)第一雷射", "       1.9Set Point(EOT Off)第一雷射", "       1.10Get Point(SOT)第一雷射", "       1.11Set Point(EOT On)第二雷射", "       1.12Set Point(EOT Off)第二雷射", "       1.13Get Point(SOT)第二雷射", "2.0功能-相機控制", "       2.1相機-初始化", "       2.2相機-取像1", "       2.2相機-取像2", "       2.3相機-關閉", "3.0功能-影像控制", "       3.1影像-初始化", "       3.2影像-更新影像", "       3.3影像-儲存影像1", "       3.3影像-儲存影像2", "4.0功能-檢測", "       4.1檢測-初始化", "      4.2浪代-浪代1", "      4.2浪代-浪代2", "      4.3檢測-量測1", "      4.3檢測-量測2", "5.0功能-雷射控制", "      5.1雷射-初始化", "      5.2雷射-寫入數值1", "      5.2雷射-寫入數值2", "      5.3雷射-寫入刀數", "      5.4雷射-讀出數值", "      5.5雷射-切換", "      5.6雷射-雷射觸發", "      5.7雷射-關閉", "6.0功能-檔案", "       6.1檔案-初始化", "       6.2檔案-儲存檔案", "       6.3檔案-開啟檔案(setting)", "       6.3檔案-開啟檔案(點檢)", "       6.3檔案-開啟檔案(近點)", "       6.4檔案-匯入檔案(近點)", "       6.4檔案-開啟檔案(雷射)", "7.0 錯誤", "8.0等待", "       8.1等待(計算時間)", "9.0離開", "10.0功能-機台驗證", "      10.1機台驗證-初始化", "      10.2機台驗證-檢測", "11.0對話視窗"]
              }
            }
          }
          frame Enabled {
          }
        }
        n67 = for {
          tunnel: w143 -> [w152]
          tunnel: w142 -> [w151]
          tunnel: [w150] -> w141
          tunnel: w139 -> [w149] mode=indexing
          tunnel: [w148] -> w140
          n68 = Enqueue Element(queue=w152, element=w149, error in (no error)=w151) -> (queue out=w150:refnum<queue>, error out=w148:errorcluster)  [unwired: 1 in, 1 out]
        }
      }
      frame "三、動作-離開" {
        w155 = T4[] [enum."       2.3相機-關閉", enum."      5.7雷射-關閉", enum."       6.2檔案-儲存檔案", enum."9.0離開"] items=["一、動作-初始化", "二、動作-連線測試", "三、動作-離開", "1.0 功能-IO控制", "       1.1 IO-初始化", "       1.2 Set Point(EOT On)第一拍照", "       1.3Set Point(EOT Off)第一拍照", "       1.4Get Point(SOT)第一拍照", "       1.5Set Point(EOT On)第二拍照", "       1.6Set Point(EOT Off)第二拍照", "       1.7Get Point(SOT)第二拍照", "       1.8Set Point(EOT On)第一雷射", "       1.9Set Point(EOT Off)第一雷射", "       1.10Get Point(SOT)第一雷射", "       1.11Set Point(EOT On)第二雷射", "       1.12Set Point(EOT Off)第二雷射", "       1.13Get Point(SOT)第二雷射", "2.0功能-相機控制", "       2.1相機-初始化", "       2.2相機-取像1", "       2.2相機-取像2", "       2.3相機-關閉", "3.0功能-影像控制", "       3.1影像-初始化", "       3.2影像-更新影像", "       3.3影像-儲存影像1", "       3.3影像-儲存影像2", "4.0功能-檢測", "       4.1檢測-初始化", "      4.2浪代-浪代1", "      4.2浪代-浪代2", "      4.3檢測-量測1", "      4.3檢測-量測2", "5.0功能-雷射控制", "      5.1雷射-初始化", "      5.2雷射-寫入數值1", "      5.2雷射-寫入數值2", "      5.3雷射-寫入刀數", "      5.4雷射-讀出數值", "      5.5雷射-切換", "      5.6雷射-雷射觸發", "      5.7雷射-關閉", "6.0功能-檔案", "       6.1檔案-初始化", "       6.2檔案-儲存檔案", "       6.3檔案-開啟檔案(setting)", "       6.3檔案-開啟檔案(點檢)", "       6.3檔案-開啟檔案(近點)", "       6.4檔案-匯入檔案(近點)", "       6.4檔案-開啟檔案(雷射)", "7.0 錯誤", "8.0等待", "       8.1等待(計算時間)", "9.0離開", "10.0功能-機台驗證", "      10.1機台驗證-初始化", "      10.2機台驗證-檢測", "11.0對話視窗"]
        n69 = for {
          tunnel: [w162] -> w157
          tunnel: [w161] -> w156
          tunnel: w155 -> [w160] mode=indexing
          tunnel: w154 -> [w159]
          tunnel: w153 -> [w158]
          n70 = Enqueue Element(queue=w159, element=w160, error in (no error)=w158) -> (queue out=w162:refnum<queue>, error out=w161:errorcluster)  [unwired: 1 in, 1 out]
        }
      }
      frame "1.0 功能-IO控制" {
      }
      frame "       1.1 IO-初始化" {
        n71 = call "量測_IO.vi"("IO_Action"=T11."Initialize") -> ()  [unwired: 9 in, 2 out]
      }
      frame "       1.2 Set Point(EOT On)第一拍照" {
        n72 = Bundle By Name(cluster=T12 {"CardID"=0, "Point#"=0, "Point Status"=FALSE, "Port"=0, "Port Status"=[]} ("IO In"), "CardID"=u8 0, "Point#"=u8 0, "Point Status"=TRUE) -> (w168:T12)
        n73 = call "量測_IO.vi"("IO_Action"=T11."Set Point", "IO In"=w168) -> ()  [unwired: 8 in, 2 out]
      }
      frame "       1.3Set Point(EOT Off)第一拍照" {
        n74 = Bundle By Name(cluster=T12 {"CardID"=0, "Point#"=0, "Point Status"=FALSE, "Port"=0, "Port Status"=[]} ("IO In"), "CardID"=u8 0, "Point#"=u8 0, "Point Status"=FALSE) -> (w176:T12)
        n75 = call "量測_IO.vi"("IO_Action"=T11."Set Point", "IO In"=w176) -> ()  [unwired: 8 in, 2 out]
      }
      frame "       1.4Get Point(SOT)第一拍照" {
        w191 = u8 0 ("CardID")
        n76 = Bundle By Name(cluster=T12 {"CardID"=0, "Point#"=0, "Point Status"=FALSE, "Port"=0, "Port Status"=[]} ("IO In"), "CardID"=w191, "Point#"=w191) -> (w192:T12)
        n77 = call "量測_IO.vi"("IO_Action"=T11."Read Point", "Error in"=w187, "IO In"=w192) -> ("Error Out"=w189:errorcluster, "IO Out"=w190:T12)  [unwired: 7 in]
        n78 = Unbundle By Name(w190) -> ("Point Status"=w184:bool)
        n79 = case shown="False" w184 {
          tunnel: w189 -> [w198 w200]
          tunnel: w188 -> [w199 w201]
          tunnel: [w197 w201] -> w186
          tunnel: [w196 w200] -> w185
          frame False {
            n80 = Enqueue Element At Opposite End(queue=w199, element=連線測試_Control_Main_Action."       1.4Get Point(SOT)第一拍照", error in (no error)=w198) -> (queue out=w197:refnum<queue>, error out=w196:errorcluster)  [unwired: 1 in, 1 out]
          }
          frame True {
          }
        }
      }
      frame "       1.5Set Point(EOT On)第二拍照" {
        n81 = Bundle By Name(cluster=T12 {"CardID"=0, "Point#"=0, "Point Status"=FALSE, "Port"=0, "Port Status"=[]} ("IO In"), "CardID"=u8 0, "Point#"=u8 1, "Point Status"=TRUE) -> (w202:T12)
        n82 = call "量測_IO.vi"("IO_Action"=T11."Set Point", "IO In"=w202) -> ()  [unwired: 8 in, 2 out]
      }
      frame "       1.6Set Point(EOT Off)第二拍照" {
        n83 = Bundle By Name(cluster=T12 {"CardID"=0, "Point#"=0, "Point Status"=FALSE, "Port"=0, "Port Status"=[]} ("IO In"), "CardID"=u8 0, "Point#"=u8 1, "Point Status"=FALSE) -> (w210:T12)
        n84 = call "量測_IO.vi"("IO_Action"=T11."Set Point", "IO In"=w210) -> ()  [unwired: 8 in, 2 out]
      }
      frame "       1.7Get Point(SOT)第二拍照" {
        n85 = Bundle By Name(cluster=T12 {"CardID"=0, "Point#"=0, "Point Status"=FALSE, "Port"=0, "Port Status"=[]} ("IO In"), "CardID"=u8 0, "Point#"=u8 1 ("CardID")) -> (w227:T12)
        n86 = call "量測_IO.vi"("IO_Action"=T11."Read Point", "Error in"=w222, "IO In"=w227) -> ("Error Out"=w221:errorcluster, "IO Out"=w225:T12)  [unwired: 7 in]
        n87 = Unbundle By Name(w225) -> ("Point Status"=w224:bool)
        n88 = case shown="False" w224 {
          tunnel: [w234 w236] -> w220
          tunnel: [w233 w235] -> w219
          tunnel: w223 -> [w231 w236]
          tunnel: w221 -> [w230 w235]
          frame False {
            n89 = Enqueue Element At Opposite End(queue=w231, element=連線測試_Control_Main_Action."       1.7Get Point(SOT)第二拍照", error in (no error)=w230) -> (queue out=w234:refnum<queue>, error out=w233:errorcluster)  [unwired: 1 in, 1 out]
          }
          frame True {
          }
        }
      }
      frame "       1.8Set Point(EOT On)第一雷射" {
        n90 = Bundle By Name(cluster=T12 {"CardID"=0, "Point#"=0, "Point Status"=FALSE, "Port"=0, "Port Status"=[]} ("IO In"), "CardID"=u8 0, "Point#"=u8 2, "Point Status"=TRUE) -> (w237:T12)
        n91 = call "量測_IO.vi"("IO_Action"=T11."Set Point", "IO In"=w237) -> ()  [unwired: 8 in, 2 out]
      }
      frame "       1.9Set Point(EOT Off)第一雷射" {
        n92 = Bundle By Name(cluster=T12 {"CardID"=0, "Point#"=0, "Point Status"=FALSE, "Port"=0, "Port Status"=[]} ("IO In"), "CardID"=u8 0, "Point#"=u8 2, "Point Status"=FALSE) -> (w245:T12)
        n93 = call "量測_IO.vi"("IO_Action"=T11."Set Point", "IO In"=w245) -> ()  [unwired: 8 in, 2 out]
      }
      frame "       1.10Get Point(SOT)第一雷射" {
        n94 = Bundle By Name(cluster=T12 {"CardID"=0, "Point#"=0, "Point Status"=FALSE, "Port"=0, "Port Status"=[]} ("IO In"), "CardID"=u8 0, "Point#"=u8 6 ("CardID")) -> (w262:T12)
        n95 = call "量測_IO.vi"("IO_Action"=T11."Read Point", "Error in"=w257, "IO In"=w262) -> ("Error Out"=w256:errorcluster, "IO Out"=w260:T12)  [unwired: 7 in]
        n96 = Unbundle By Name(w260) -> ("Point Status"=w259:bool)
        n97 = case shown="False" w259 {
          tunnel: [w269 w271] -> w255
          tunnel: [w268 w270] -> w254
          tunnel: w258 -> [w266 w271]
          tunnel: w256 -> [w265 w270]
          frame False {
            n98 = Enqueue Element At Opposite End(queue=w266, element=連線測試_Control_Main_Action."       1.10Get Point(SOT)第一雷射", error in (no error)=w265) -> (queue out=w269:refnum<queue>, error out=w268:errorcluster)  [unwired: 1 in, 1 out]
          }
          frame True {
          }
        }
      }
      frame "       1.11Set Point(EOT On)第二雷射" {
        n99 = Bundle By Name(cluster=T12 {"CardID"=0, "Point#"=0, "Point Status"=FALSE, "Port"=0, "Port Status"=[]} ("IO In"), "CardID"=u8 0, "Point#"=u8 3, "Point Status"=TRUE) -> (w273:T12)
        n100 = call "量測_IO.vi"("IO_Action"=T11."Set Point", "IO In"=w273) -> ()  [unwired: 8 in, 2 out]
        n101 = Wait (ms)(milliseconds to wait=u32 1000) -> ()  [unwired: 1 out]
      }
      frame "       1.12Set Point(EOT Off)第二雷射" {
        n102 = Bundle By Name(cluster=T12 {"CardID"=0, "Point#"=0, "Point Status"=FALSE, "Port"=0, "Port Status"=[]} ("IO In"), "CardID"=u8 0, "Point#"=u8 3, "Point Status"=FALSE) -> (w281:T12)
        n103 = call "量測_IO.vi"("IO_Action"=T11."Set Point", "IO In"=w281) -> ()  [unwired: 8 in, 2 out]
      }
      frame "       1.13Get Point(SOT)第二雷射" {
        n104 = Bundle By Name(cluster=T12 {"CardID"=0, "Point#"=0, "Point Status"=FALSE, "Port"=0, "Port Status"=[]} ("IO In"), "CardID"=u8 0, "Point#"=u8 7 ("CardID")) -> (w298:T12)
        n105 = call "量測_IO.vi"("IO_Action"=T11."Read Point", "Error in"=w293, "IO In"=w298) -> ("Error Out"=w292:errorcluster, "IO Out"=w296:T12)  [unwired: 7 in]
        n106 = Unbundle By Name(w296) -> ("Point Status"=w295:bool)
        n107 = case shown="False" w295 {
          tunnel: [w305 w307] -> w291
          tunnel: [w304 w306] -> w290
          tunnel: w294 -> [w302 w307]
          tunnel: w292 -> [w301 w306]
          frame False {
            n108 = Enqueue Element At Opposite End(queue=w302, element=連線測試_Control_Main_Action."       1.13Get Point(SOT)第二雷射", error in (no error)=w301) -> (queue out=w305:refnum<queue>, error out=w304:errorcluster)  [unwired: 1 in, 1 out]
          }
          frame True {
          }
        }
      }
      frame "2.0功能-相機控制" {
      }
      frame "       2.1相機-初始化" {
        n109 = call "cameraFGV.vi"("action_camera"=action_camera."初始化", "Session In"=w310) -> ()  [unwired: 7 in, 3 out]
      }
      frame "       2.2相機-取像1" {
        n110 = case shown="True" w314 {
          tunnel: w317 -> [w327 _]
          frame False {
            n111 = call "Image FGV.vi"("Image action"=Image_action."讀取圖片", "圖片名稱"="Image_1") -> ("error out"=w323:errorcluster, "Image Out"=w324:T3)  [unwired: 8 in]
            n112 = call "cameraFGV.vi"("action_camera"=action_camera."取像", "error constant"=w323, "Image In"=w324, "Session In"=w327) -> ("error constant 2"=w322:errorcluster, "Image Out"=w321:T3)  [unwired: 5 in, 1 out]
            n113 = call "Image FGV.vi"("Image action"=Image_action."寫入圖片", "error in (no error)"=w322, "Image In"=w321, "圖片名稱"="Image_1") -> ()  [unwired: 6 in, 2 out]
          }
          frame True {
            n114 = call "Image FGV.vi"("Image action"=Image_action."讀取圖片", "圖片名稱"="Image_1") -> ("error out"=w329:errorcluster, "Image Out"=w330:T3)  [unwired: 8 in]
            n115 = call "IMAQ Load Image Dialog"() -> ("Path"=w328:path)  [unwired: 9 in, 2 out]
            n116 = call "IMAQ ReadFile"("File Path"=w328, "error in (no error)"=w329, "Image"=w330) -> ()  [unwired: 4 in, 5 out]
          }
        }
      }
      frame "       2.2相機-取像2" {
        n117 = case shown="True" w334 {
          tunnel: w333 -> [w337 _]
          frame False {
            n118 = call "Image FGV.vi"("Image action"=Image_action."讀取圖片", "圖片名稱"="Image_2") -> ("error out"=w343:errorcluster, "Image Out"=w344:T3)  [unwired: 8 in]
            n119 = call "cameraFGV.vi"("action_camera"=action_camera."取像", "error constant"=w343, "Image In"=w344, "Session In"=w337) -> ("error constant 2"=w342:errorcluster, "Image Out"=w341:T3)  [unwired: 5 in, 1 out]
            n120 = call "Image FGV.vi"("Image action"=Image_action."寫入圖片", "error in (no error)"=w342, "Image In"=w341, "圖片名稱"="Image_2") -> ()  [unwired: 6 in, 2 out]
          }
          frame True {
            n121 = call "Image FGV.vi"("Image action"=Image_action."讀取圖片", "圖片名稱"="Image_2") -> ("error out"=w348:errorcluster, "Image Out"=w349:T3)  [unwired: 8 in]
            n122 = call "IMAQ Load Image Dialog"() -> ("Path"=w347:path)  [unwired: 9 in, 2 out]
            n123 = call "IMAQ ReadFile"("File Path"=w347, "error in (no error)"=w348, "Image"=w349) -> ()  [unwired: 4 in, 5 out]
          }
        }
      }
      frame "       2.3相機-關閉" {
        n124 = call "cameraFGV.vi"("action_camera"=action_camera."結束", "Session In"=w352) -> ()  [unwired: 7 in, 3 out]
      }
      frame "3.0功能-影像控制" {
      }
      frame "       3.1影像-初始化" {
        w358 = T35[] [0, 0, 0, 0] items=["Grayscale (U8)", "Grayscale (I16)", "Grayscale (SGL)", "Complex (CSG)", "RGB (U32)", "HSL (U32)", "RGB (U64)", "Grayscale (U16)"]
        n125 = call "Image FGV.vi"("Image action"=Image_action."初始化") -> ("error out"=w360:errorcluster)  [unwired: 9 in, 1 out]
        n126 = for {
          tunnel: w360 -> [w367]
          tunnel: string[] ["Image_1", "Pattern_L", "Pattern_R", "Image_2"] -> [w365] mode=indexing
          tunnel: w358 -> [w364] mode=indexing
          n127 = call "Image FGV.vi"("Image action"=Image_action."創造記憶體", "error in (no error)"=w367, "Image Type"=w364, "圖片名稱"=w365) -> ()  [unwired: 6 in, 2 out]
        }
      }
      frame "       3.2影像-更新影像" {
        n128 = call "Image FGV.vi"("Image action"=Image_action."讀取圖片", "圖片名稱"="Image_1") -> ("error out"=w379:errorcluster, "Image Out"=w378:T3)  [unwired: 8 in]
        n129 = call "Image FGV.vi"("Image action"=Image_action."讀取圖片", "圖片名稱"="Image_2") -> ("error out"=w376:errorcluster, "Image Out"=w377:T3)  [unwired: 8 in]
        n130 = call "Image FGV.vi"("Image action"=Image_action."讀取圖片", "圖片名稱"="Pattern_L") -> ("Image Out"=→"Patttern_L":T3)  [unwired: 8 in, 1 out]
        n131 = call "Image FGV.vi"("Image action"=Image_action."讀取圖片", "圖片名稱"="Pattern_R") -> ("Image Out"=→"Patttern_R":T3)  [unwired: 8 in, 1 out]
        n132 = call "點檢_VI_畫十字線.vi"("error in (no error)"=w379, "Refnum in"=w378) -> ("error out"=w375:errorcluster, "Refnum out"=w374:T3)  [unwired: 7 in, 1 out]
        n133 = call "點檢_VI_畫十字線.vi"("error in (no error)"=w376, "Refnum in"=w377) -> ("error out"=w371:errorcluster, "Refnum out"=w370:T3)  [unwired: 7 in, 1 out]
        n134 = disable-structure shown="Enabled" {
          disable-tunnel: w375 -> [w406 w408]
          disable-tunnel: w374 -> [w405 w409]
          disable-tunnel: [w404 w409] -> w373
          disable-tunnel: [w403 w408] -> w372
          frame Disabled {
            n135 = call "IMAQ BCGLookup"("Image Src"=w405, "BCG Values"=T15 {"Brightness"=128.0, "Contrast"=84.5, "Gamma"=1.0}, "error in (no error)"=w406) -> ("Image Dst Out"=w404:T3, "error out"=w403:errorcluster)  [unwired: 4 in]
          }
          frame Enabled {
          }
        }
        "Image1" <- w373
        n136 = disable-structure shown="Enabled" {
          disable-tunnel: w371 -> [w399 w401]
          disable-tunnel: w370 -> [w398 w402]
          disable-tunnel: [w397 w402] -> w369
          disable-tunnel: [w396 w401] -> w368
          frame Disabled {
            n137 = call "IMAQ BCGLookup"("Image Src"=w398, "BCG Values"=T15 {"Brightness"=128.0, "Contrast"=84.5, "Gamma"=1.0}, "error in (no error)"=w399) -> ("Image Dst Out"=w397:T3, "error out"=w396:errorcluster)  [unwired: 4 in]
          }
          frame Enabled {
          }
        }
        "Image 2" <- w369
        n138 = property on="Image 2" class="ImageControl"("Zoom to Fit Mode"=TRUE) -> ()  [unwired: 2 in, 2 out]
        n139 = property on="Image1" class="ImageControl"("Zoom to Fit Mode"=TRUE) -> ()  [unwired: 2 in, 2 out]
        n140 = property on="Patttern_L" class="ImageControl"("Zoom to Fit Mode"=TRUE) -> ()  [unwired: 2 in, 2 out]
        n141 = property on="Patttern_R" class="ImageControl"("Zoom to Fit Mode"=TRUE) -> ()  [unwired: 2 in, 2 out]
      }
      frame "       3.3影像-儲存影像1" {
        n142 = case shown="True" w414 {
          tunnel: w413 -> [w415 w419]
          tunnel: [w415 w418] -> w410
          tunnel: w412 -> [w416 w417]
          tunnel: [w416 w417] -> w411
          frame False {
          }
          frame True {
            n143 = call "Image FGV.vi"("Image action"=Image_action."讀取圖片", "圖片名稱"="Image_1") -> ("Image Out"=w426:T3)  [unwired: 8 in, 1 out]
            n144 = Format Date/Time String(time format string (%c)="%Y-%m-%d-%H-%M-%S-%2u") -> (date/time string=w421:string)  [unwired: 2 in]
            n145 = Concatenate Strings(w421, ".png" ("string")) -> (w422:string)
            n146 = Build Path(base path=path "D:/圖片", name or relative path=w422) -> (appended path=w425:path)
            n147 = call-poly "IMAQ Write File 2"("error in (no error)"=w419, "File Path"=w425, "Image"=w426) -> ("error out"=w418:errorcluster)  [unwired: 7 in, 1 out]
          }
        }
      }
      frame "       3.3影像-儲存影像2" {
        n148 = case shown="True" w433 {
          tunnel: w432 -> [w435 w438]
          tunnel: [w435 w438] -> w430
          tunnel: w431 -> [w434 w437]
          tunnel: [w434 w436] -> w429
          frame False {
          }
          frame True {
            n149 = call "Image FGV.vi"("Image action"=Image_action."讀取圖片", "圖片名稱"="Image_2") -> ("Image Out"=w445:T3)  [unwired: 8 in, 1 out]
            n150 = Format Date/Time String(time format string (%c)="%Y-%m-%d-%H-%M-%S-%2u") -> (date/time string=w440:string)  [unwired: 2 in]
            n151 = Concatenate Strings(w440, ".png" ("string")) -> (w439:string)
            n152 = Build Path(base path=path "D:/", name or relative path=w439) -> (appended path=w443:path)
            n153 = call-poly "IMAQ Write File 2"("error in (no error)"=w437, "File Path"=w443, "Image"=w445) -> ("error out"=w436:errorcluster)  [unwired: 7 in, 1 out]
          }
        }
      }
      frame "4.0功能-檢測" {
      }
      frame "       4.1檢測-初始化" {
      }
      frame "      4.2浪代-浪代1" {
        w458 = "邊R座標-1"
        w462 = "邊L座標-1"
        w499 = u16 1 items=["Find Reference", "Update CoordSys"] ("Mode")
        w509 = u16 1 items=["Find Reference", "Update CoordSys"] ("Mode")
        # "Match與找邊setting參數"
        n154 = for {
          tunnel: [w515] -> w455 mode=indexing
          tunnel: string[] ["Match_L", "Match_R", "找邊_L", "找邊R"] -> [w514] mode=indexing
          n155 = call "Main_FGV_Data.vi"("Action_Data"=Action_Data."Get Data", "Data name"=w514) -> ("Data  Out"=w515:cluster{"Data name":string, "Data":variant})  [unwired: 8 in, 1 out]
        }
        n156 = Index Array(array=w455, index #1=0 ("index"), index #2=1 ("index"), index #3=2 ("index"), index #4=3 ("index")) -> (element #1=w504:cluster{"Data name":string, "Data":variant}, element #2=w497:cluster{"Data name":string, "Data":variant}, element #3=w488:cluster{"Data name":string, "Data":variant}, element #4=w475:cluster{"Data name":string, "Data":variant})
        n157 = call "Image FGV.vi"("Image action"=Image_action."讀取圖片", "圖片名稱"="Image_1") -> ("error out"=w456:errorcluster, "Image Out"=w492:T3)  [unwired: 8 in]
        n158 = Unbundle By Name(w504) -> ("Data"=w503:variant)
        n159 = Unbundle By Name(w497) -> ("Data"=w496:variant)
        n160 = Unbundle By Name(w488) -> ("Data"=w487:variant)
        n161 = Unbundle By Name(w475) -> ("Data"=w473:variant)
        n162 = call "Image FGV.vi"("Image action"=Image_action."讀取圖片", "圖片名稱"="Pattern_L") -> ("Image Out"=w508:T3)  [unwired: 8 in, 1 out]
        n163 = Variant To Data(type=T24 {"樣本比對參數L"={"方法"=0, "分數"=0.0, "起始角度"=0.0, "結束角度"=0.0}, "ROI"={"Global Rectangle"=[], "Contours"=[]}, "Coordinate System Out"={"Reference System"={"Origin"={"X"=0.0, "Y"=0.0}, "Angle (deg)"=0.0, "Axis Reference"=0}, "Measurement System"={"Origin"={"X"=0.0, "Y"=0.0}, "Angle (deg)"=0.0, "Axis Reference"=0}}} ("output cluster"), Variant=w503) -> (data=w507:T24)  [unwired: 1 in, 1 out]
        n164 = Variant To Data(type=T19 {"邊參數R"={"Search Direction"=0, "Edge Polarity"=0, "Kernel Size"=0, "Width"=0, "Minimum Edge Strength"=0.0}, "ROI"={"Global Rectangle"=[], "Contours"=[]}} ("output cluster"), Variant=w473) -> (data=w470:T19)  [unwired: 1 in, 1 out]
        n165 = Variant To Data(type=T20 {"邊參數L"={"Search Direction"=0, "Edge Polarity"=0, "Kernel Size"=0, "Width"=0, "Minimum Edge Strength"=0.0}, "ROI"={"Global Rectangle"=[], "Contours"=[]}} ("output cluster"), Variant=w487) -> (data=w486:T20)  [unwired: 1 in, 1 out]
        n166 = Unbundle(w507) -> ("樣本比對參數L"=w481:T21, "ROI"=w506:T36, "Coordinate System Out"=w483:T22)
        n167 = call "浪代_Match_Sub.vi"("樣本比對參數"=w481, "ROI Descriptor"=w506, "Mode"=w509, "error in (no error)"=w456, "Coordinate System In"=w483, "Template Image"=w508, "Image"=w492) -> ("error out"=w498:errorcluster, "Coordinate System Out"=w484:T22)  [unwired: 2 in, 1 out]
        n168 = Variant To Data(type=T23 {"ROI"={"Global Rectangle"=[], "Contours"=[]}, "樣本比對參數R"={"方法"=0, "分數"=0.0, "起始角度"=0.0, "結束角度"=0.0}, "Coordinate System Out"={"Reference System"={"Origin"={"X"=0.0, "Y"=0.0}, "Angle (deg)"=0.0, "Axis Reference"=0}, "Measurement System"={"Origin"={"X"=0.0, "Y"=0.0}, "Angle (deg)"=0.0, "Axis Reference"=0}}} ("output cluster"), Variant=w496) -> (data=w495:T23)  [unwired: 1 in, 1 out]
        n169 = Unbundle(w470) -> ("邊參數R"=w468:T17, "ROI"=w469:T36)
        n170 = Unbundle(w486) -> ("邊參數L"=w477:T17, "ROI"=w485:T36)
        n171 = Unbundle(w495) -> ("ROI"=w494:T36, "樣本比對參數R"=w479:T21, "Coordinate System Out"=w493:T22)
        n172 = call "Image FGV.vi"("Image action"=Image_action."讀取圖片", "圖片名稱"="Pattern_R") -> ("Image Out"=w500:T3)  [unwired: 8 in, 1 out]
        n173 = call "浪代_Match_Sub.vi"("樣本比對參數"=w479, "ROI Descriptor"=w494, "Mode"=w499, "error in (no error)"=w498, "Coordinate System In"=w493, "Template Image"=w500, "Image"=w492) -> ("error out"=w476:errorcluster, "Coordinate System Out"=w467:T22)  [unwired: 2 in, 1 out]
        n174 = call "浪代_Line_Sub.vi"("邊參數"=w477, "error in (no error)"=w476, "ROI"=w485, "Coordinate System"=w484, "Image"=w492) -> ("error out"=w472:errorcluster, "線段2端點"=w465:T26, "Image Out"=w471:T3)  [unwired: 4 in]
        n175 = call "浪代_Line_Sub.vi"("邊參數"=w468, "error in (no error)"=w472, "ROI"=w469, "Coordinate System"=w467, "Image"=w471) -> ("線段2端點"=w457:T26)  [unwired: 4 in, 2 out]
        n176 = To Variant(anything=w457) -> (Variant=w460:variant)
        n177 = To Variant(anything=w465) -> (Variant=w464:variant)
        n178 = Bundle(w458, "Variant"=w460) -> (w459:cluster{string, "Variant":variant})  [unwired: 1 in]
        n179 = Bundle(w462, "Variant"=w464) -> (w463:cluster{string, "Variant":variant})  [unwired: 1 in]
        n180 = call "Main_FGV_Data.vi"("Action_Data"=Action_Data."Set Data", "Data In"=w459, "Data name"=w458) -> ()  [unwired: 7 in, 2 out]
        n181 = call "Main_FGV_Data.vi"("Action_Data"=Action_Data."Set Data", "Data In"=w463, "Data name"=w462) -> ()  [unwired: 7 in, 2 out]
      }
      frame "      4.2浪代-浪代2" {
        w523 = "邊R座標"
        w527 = "邊L座標"
        w564 = u16 1 items=["Find Reference", "Update CoordSys"] ("Mode")
        w574 = u16 1 items=["Find Reference", "Update CoordSys"] ("Mode")
        # "Match與找邊setting參數"
        n182 = for {
          tunnel: [w580] -> w520 mode=indexing
          tunnel: string[] ["Match_L", "Match_R", "找邊_L", "找邊R"] -> [w579] mode=indexing
          n183 = call "Main_FGV_Data.vi"("Action_Data"=Action_Data."Get Data", "Data name"=w579) -> ("Data  Out"=w580:cluster{"Data name":string, "Data":variant})  [unwired: 8 in, 1 out]
        }
        n184 = call "Image FGV.vi"("Image action"=Image_action."讀取圖片", "圖片名稱"="Image_2") -> ("error out"=w521:errorcluster, "Image Out"=w557:T3)  [unwired: 8 in]
        n185 = Index Array(array=w520, index #1=0 ("index"), index #2=1 ("index"), index #3=2 ("index"), index #4=3 ("index")) -> (element #1=w569:cluster{"Data name":string, "Data":variant}, element #2=w562:cluster{"Data name":string, "Data":variant}, element #3=w553:cluster{"Data name":string, "Data":variant}, element #4=w540:cluster{"Data name":string, "Data":variant})
        n186 = Unbundle By Name(w569) -> ("Data"=w568:variant)
        n187 = Unbundle By Name(w562) -> ("Data"=w561:variant)
        n188 = Unbundle By Name(w553) -> ("Data"=w552:variant)
        n189 = Unbundle By Name(w540) -> ("Data"=w538:variant)
        n190 = call "Image FGV.vi"("Image action"=Image_action."讀取圖片", "圖片名稱"="Pattern_L") -> ("Image Out"=w573:T3)  [unwired: 8 in, 1 out]
        n191 = Variant To Data(type=T24 {"樣本比對參數L"={"方法"=0, "分數"=0.0, "起始角度"=0.0, "結束角度"=0.0}, "ROI"={"Global Rectangle"=[], "Contours"=[]}, "Coordinate System Out"={"Reference System"={"Origin"={"X"=0.0, "Y"=0.0}, "Angle (deg)"=0.0, "Axis Reference"=0}, "Measurement System"={"Origin"={"X"=0.0, "Y"=0.0}, "Angle (deg)"=0.0, "Axis Reference"=0}}} ("output cluster"), Variant=w568) -> (data=w572:T24)  [unwired: 1 in, 1 out]
        n192 = Variant To Data(type=T19 {"邊參數R"={"Search Direction"=0, "Edge Polarity"=0, "Kernel Size"=0, "Width"=0, "Minimum Edge Strength"=0.0}, "ROI"={"Global Rectangle"=[], "Contours"=[]}} ("output cluster"), Variant=w538) -> (data=w535:T19)  [unwired: 1 in, 1 out]
        n193 = Variant To Data(type=T20 {"邊參數L"={"Search Direction"=0, "Edge Polarity"=0, "Kernel Size"=0, "Width"=0, "Minimum Edge Strength"=0.0}, "ROI"={"Global Rectangle"=[], "Contours"=[]}} ("output cluster"), Variant=w552) -> (data=w551:T20)  [unwired: 1 in, 1 out]
        n194 = Unbundle(w572) -> ("樣本比對參數L"=w546:T21, "ROI"=w571:T36, "Coordinate System Out"=w548:T22)
        n195 = call "浪代_Match_Sub.vi"("樣本比對參數"=w546, "ROI Descriptor"=w571, "Mode"=w574, "error in (no error)"=w521, "Coordinate System In"=w548, "Template Image"=w573, "Image"=w557) -> ("error out"=w563:errorcluster, "Coordinate System Out"=w549:T22)  [unwired: 2 in, 1 out]
        n196 = Variant To Data(type=T23 {"ROI"={"Global Rectangle"=[], "Contours"=[]}, "樣本比對參數R"={"方法"=0, "分數"=0.0, "起始角度"=0.0, "結束角度"=0.0}, "Coordinate System Out"={"Reference System"={"Origin"={"X"=0.0, "Y"=0.0}, "Angle (deg)"=0.0, "Axis Reference"=0}, "Measurement System"={"Origin"={"X"=0.0, "Y"=0.0}, "Angle (deg)"=0.0, "Axis Reference"=0}}} ("output cluster"), Variant=w561) -> (data=w560:T23)  [unwired: 1 in, 1 out]
        n197 = Unbundle(w535) -> ("邊參數R"=w533:T17, "ROI"=w534:T36)
        n198 = Unbundle(w551) -> ("邊參數L"=w542:T17, "ROI"=w550:T36)
        n199 = Unbundle(w560) -> ("ROI"=w559:T36, "樣本比對參數R"=w544:T21, "Coordinate System Out"=w558:T22)
        n200 = call "Image FGV.vi"("Image action"=Image_action."讀取圖片", "圖片名稱"="Pattern_R") -> ("Image Out"=w565:T3)  [unwired: 8 in, 1 out]
        n201 = call "浪代_Match_Sub.vi"("樣本比對參數"=w544, "ROI Descriptor"=w559, "Mode"=w564, "error in (no error)"=w563, "Coordinate System In"=w558, "Template Image"=w565, "Image"=w557) -> ("error out"=w541:errorcluster, "Coordinate System Out"=w532:T22)  [unwired: 2 in, 1 out]
        n202 = call "浪代_Line_Sub.vi"("邊參數"=w542, "error in (no error)"=w541, "ROI"=w550, "Coordinate System"=w549, "Image"=w557) -> ("error out"=w537:errorcluster, "線段2端點"=w530:T26, "Image Out"=w536:T3)  [unwired: 4 in]
        n203 = call "浪代_Line_Sub.vi"("邊參數"=w533, "error in (no error)"=w537, "ROI"=w534, "Coordinate System"=w532, "Image"=w536) -> ("線段2端點"=w522:T26)  [unwired: 4 in, 2 out]
        n204 = To Variant(anything=w522) -> (Variant=w525:variant)
        n205 = To Variant(anything=w530) -> (Variant=w529:variant)
        n206 = Bundle(w523, "Variant"=w525) -> (w524:cluster{string, "Variant":variant})  [unwired: 1 in]
        n207 = Bundle(w527, "Variant"=w529) -> (w528:cluster{string, "Variant":variant})  [unwired: 1 in]
        n208 = call "Main_FGV_Data.vi"("Action_Data"=Action_Data."Set Data", "Data In"=w524, "Data name"=w523) -> ()  [unwired: 7 in, 2 out]
        n209 = call "Main_FGV_Data.vi"("Action_Data"=Action_Data."Set Data", "Data In"=w528, "Data name"=w527) -> ()  [unwired: 7 in, 2 out]
      }
      frame "      4.3檢測-量測1" {
        w603 = "量測1"
        # "邊L與R是檢測完的邊座標\nData和找圓是點檢的值"
        n210 = for {
          tunnel: [w627] -> w622 mode=indexing
          tunnel: string[] ["邊L座標-1", "邊R座標-1", "Dataオ", "找圓左"] -> [w626] mode=indexing
          n211 = call "Main_FGV_Data.vi"("Action_Data"=Action_Data."Get Data", "Data name"=w626) -> ("Data  Out"=w627:cluster{"Data name":string, "Data":variant})  [unwired: 8 in, 1 out]
        }
        n212 = Index Array(array=w622, index #1=0 ("index"), index #2=1 ("index"), index #3=2 ("index"), index #4=3 ("index")) -> (element #1=w619:cluster{"Data name":string, "Data":variant}, element #2=w615:cluster{"Data name":string, "Data":variant}, element #3=w611:cluster{"Data name":string, "Data":variant}, element #4=w608:cluster{"Data name":string, "Data":variant})
        n213 = Unbundle By Name(w608) -> ("Data"=w607:variant)
        n214 = Unbundle By Name(w619) -> ("Data"=w617:variant)
        n215 = Unbundle By Name(w611) -> ("Data"=w613:variant)
        n216 = Unbundle By Name(w615) -> ("Data"=w614:variant)
        n217 = Variant To Data(type=T26 {"點1 (Pixels)"={"X"=0.0, "Y"=0.0}, "點2 (Pixels)"={"X"=0.0, "Y"=0.0}, "Angle (Pixel)"=0.0} ("線段2端點"), Variant=w617) -> (data=w589:T26)  [unwired: 1 in, 1 out]
        n218 = Variant To Data(type=T26 {"點1 (Pixels)"={"X"=0.0, "Y"=0.0}, "點2 (Pixels)"={"X"=0.0, "Y"=0.0}, "Angle (Pixel)"=0.0} ("線段2端點"), Variant=w614) -> (data=w588:T26)  [unwired: 1 in, 1 out]
        n219 = Variant To Data(type=T25 {"ROI"={"Global Rectangle"=[], "Contours"=[]}, "圓心 (Pixels)"={"X"=0.0, "Y"=0.0}} ("output cluster"), Variant=w607) -> (data=w605:T25)  [unwired: 1 in, 1 out]
        n220 = Variant To Data(type=cluster{sgl, sgl} {0.0, 0.0} ("x-y"), Variant=w613) -> (data=w591:cluster{sgl, sgl})  [unwired: 1 in, 1 out]
        n221 = Unbundle By Name(w605) -> ("圓心 (Pixels)"=w590:cluster{"X":sgl, "Y":sgl})
        n222 = call "Image FGV.vi"("Image action"=Image_action."讀取圖片", "圖片名稱"="Image_1") -> ("Image Out"=w597:T3)  [unwired: 8 in, 1 out]
        n223 = local read "總值左out"() -> (w594:dbl)
        n224 = local read "總值右out"() -> (w593:dbl)
        n225 = Bundle("總值左out"=w594, "總值右out"=w593) -> (w587:cluster{"總值左out":dbl, "總值右out":dbl})  [unwired: 1 in]
        n226 = call "量測_VI_Offect2.vi"("Image"=w597, "pixel轉mm"="pixel轉mm(左)", "data"=w591, "圓心 (Pixels)"=w590, "左邊座標"=w589, "右邊座標"=w588, "offect總值 in"=w587) -> ("左X分量"=w586:dbl, "左Y分量"=w585:dbl, "右X分量"=w584:dbl, "右Y分量"=w583:dbl, "offect總值 out"=w592:cluster{"總值左out":dbl, "總值右out ":dbl})  [unwired: 4 in]
        n227 = Unbundle(w592) -> ("總值左out"=→"總值左out":dbl, "總值右out"=→"總值右out":dbl)
        n228 = Bundle("左X分量"=w586, "左Y分量"=w585, "右X分量"=w584, "右Y分量"=w583, "pixel轉mm(左)"="pixel轉mm(左)", "offect總值 out"=w592) -> (w602:T29)  [unwired: 1 in]
        n229 = To Variant(anything=w602) -> (Variant=w601:variant)
        n230 = Bundle(w603, "Variant"=w601) -> (w600:cluster{string, "Variant":variant})  [unwired: 1 in]
        n231 = call "Main_FGV_Data.vi"("Action_Data"=Action_Data."Set Data", "Data In"=w600, "Data name"=w603) -> ()  [unwired: 7 in, 2 out]
      }
      frame "      4.3檢測-量測2" {
        w646 = "量測2"
        # "邊L與R是檢測完的邊座標\nData和找圓是點檢的值"
        n232 = for {
          tunnel: [w674] -> w667 mode=indexing
          tunnel: string[] ["邊L座標", "邊R座標", "Data右", "找圓右"] -> [w673] mode=indexing
          n233 = call "Main_FGV_Data.vi"("Action_Data"=Action_Data."Get Data", "Data name"=w673) -> ("Data  Out"=w674:cluster{"Data name":string, "Data":variant})  [unwired: 8 in, 1 out]
        }
        n234 = Index Array(array=w667, index #1=0 ("index"), index #2=1 ("index"), index #3=2 ("index"), index #4=3 ("index")) -> (element #1=w664:cluster{"Data name":string, "Data":variant}, element #2=w661:cluster{"Data name":string, "Data":variant}, element #3=w670:cluster{"Data name":string, "Data":variant}, element #4=w653:cluster{"Data name":string, "Data":variant})
        n235 = Unbundle By Name(w664) -> ("Data"=w663:variant)
        n236 = Unbundle By Name(w653) -> ("Data"=w656:variant)
        n237 = Unbundle By Name(w670) -> ("Data"=w659:variant)
        n238 = Unbundle By Name(w661) -> ("Data"=w660:variant)
        n239 = Variant To Data(type=T26 {"點1 (Pixels)"={"X"=0.0, "Y"=0.0}, "點2 (Pixels)"={"X"=0.0, "Y"=0.0}, "Angle (Pixel)"=0.0} ("線段2端點"), Variant=w663) -> (data=w649:T26)  [unwired: 1 in, 1 out]
        n240 = Variant To Data(type=T26 {"點1 (Pixels)"={"X"=0.0, "Y"=0.0}, "點2 (Pixels)"={"X"=0.0, "Y"=0.0}, "Angle (Pixel)"=0.0} ("線段2端點"), Variant=w660) -> (data=w648:T26)  [unwired: 1 in, 1 out]
        n241 = Variant To Data(type=T25 {"ROI"={"Global Rectangle"=[], "Contours"=[]}, "圓心 (Pixels)"={"X"=0.0, "Y"=0.0}} ("output cluster"), Variant=w656) -> (data=w654:T25)  [unwired: 1 in, 1 out]
        n242 = Variant To Data(type=cluster{sgl, sgl} {0.0, 0.0} ("x-y"), Variant=w659) -> (data=w650:cluster{sgl, sgl})  [unwired: 1 in, 1 out]
        n243 = local read "總值左out 2"() -> (w632:dbl)
        n244 = local read "總值右out 2"() -> (w631:dbl)
        n245 = Unbundle By Name(w654) -> ("圓心 (Pixels)"=w651:cluster{"X":sgl, "Y":sgl})
        n246 = call "Image FGV.vi"("Image action"=Image_action."讀取圖片", "圖片名稱"="Image_2") -> ("Image Out"=w636:T3)  [unwired: 8 in, 1 out]
        n247 = Bundle("總值左out 2"=w632, "總值右out 2"=w631) -> (w630:cluster{"總值左out 2":dbl, "總值右out 2":dbl})  [unwired: 1 in]
        n248 = call "量測_VI_Offect.vi"("Image"=w636, "pixel轉mm"="pixel轉mm(右)", "data"=w650, "圓心 (Pixels)"=w651, "左邊座標"=w649, "右邊座標"=w648, "offect總值 in"=w630) -> ("左X分量"=w643:dbl, "左Y分量"=w642:dbl, "右X分量"=w641:dbl, "右Y分量"=w640:dbl, "offect總值 out"=w634:cluster{"總值左out":dbl, "總值右out ":dbl})  [unwired: 4 in]
        n249 = Unbundle(w634) -> ("總值左out"=→"總值左out 2":dbl, "總值右out"=→"總值右out 2":dbl)
        n250 = Bundle("左X分量"=w643, "左Y分量"=w642, "右X分量"=w641, "右Y分量"=w640, "pixel轉mm(右)"="pixel轉mm(右)", "offect總值 out"=w634) -> (w639:T30)  [unwired: 1 in]
        n251 = To Variant(anything=w639) -> (Variant=w645:variant)
        n252 = Bundle(w646, "Variant"=w645) -> (w644:cluster{string, "Variant":variant})  [unwired: 1 in]
        n253 = call "Main_FGV_Data.vi"("Action_Data"=Action_Data."Set Data", "Data In"=w644, "Data name"=w646) -> ()  [unwired: 7 in, 2 out]
      }
      frame "5.0功能-雷射控制" {
      }
      frame "      5.1雷射-初始化" {
        n254 = call "RS232 Device.vi"() -> ("error out"=w679:errorcluster, "COM"=w680:refnum<visa-resource-name>)  [unwired: 10 in]
        n255 = call "雷射_FGV.vi"("Enum"=T27."RS232_Init ", "error in"=w679, "VISA resource name"=w680) -> ()  [unwired: 6 in, 3 out]
      }
      frame "      5.2雷射-寫入數值1" {
        n256 = for {
          tunnel: [w786] -> w714 mode=indexing
          tunnel: string[] ["邊L座標-1", "邊R座標-1", "量測1"] -> [w785] mode=indexing
          n257 = call "Main_FGV_Data.vi"("Action_Data"=Action_Data."Get Data", "Data name"=w785) -> ("Data  Out"=w786:cluster{"Data name":string, "Data":variant})  [unwired: 8 in, 1 out]
        }
        n258 = call "Main_FGV_Data.vi"("Action_Data"=Action_Data."Get Data", "Data name"="量測1") -> ("Data  Out"=w725:cluster{"Data name":string, "Data":variant})  [unwired: 8 in, 1 out]
        n259 = Unbundle By Name(w725) -> ("Data"=w724:variant)
        n260 = call "Main_FGV_Data.vi"("Action_Data"=Action_Data."Get Data", "Data name"="參數設定") -> ("Data  Out"=w692:cluster{"Data name":string, "Data":variant})  [unwired: 8 in, 1 out]
        n261 = Index Array(array=w714, index #1=0 ("index"), index #2=1 ("index"), index #3=2 ("index")) -> (element #1=w711:cluster{"Data name":string, "Data":variant}, element #2=w707:cluster{"Data name":string, "Data":variant}, element #3=w716:cluster{"Data name":string, "Data":variant})
        n262 = Variant To Data(type=T29 {"左X分量"=0.0, "左Y分量"=0.0, "右X分量"=0.0, "右Y分量"=0.0, "pixel轉mm(左)"=0.0, "offect總值 out"={"總值左out"=0.0, "總值右out "=0.0}} ("output cluster"), Variant=w724) -> (data=w723:T29)  [unwired: 1 in, 1 out]
        n263 = Unbundle By Name(w692) -> ("Data"=w691:variant)
        n264 = Unbundle By Name(w711) -> ("Data"=w709:variant)
        n265 = Unbundle By Name(w707) -> ("Data"=w706:variant)
        n266 = Unbundle By Name(w716) -> ("Data"=w717:variant)
        n267 = Unbundle By Name(w723) -> ("左X分量"=w685:dbl, "左Y分量"=w684:dbl, "右X分量"=w686:dbl, "右Y分量"=w683:dbl)
        n268 = Variant To Data(type=T26 {"點1 (Pixels)"={"X"=0.0, "Y"=0.0}, "點2 (Pixels)"={"X"=0.0, "Y"=0.0}, "Angle (Pixel)"=0.0} ("線段2端點"), Variant=w709) -> (data=w720:T26)  [unwired: 1 in, 1 out]
        n269 = Variant To Data(type=T26 {"點1 (Pixels)"={"X"=0.0, "Y"=0.0}, "點2 (Pixels)"={"X"=0.0, "Y"=0.0}, "Angle (Pixel)"=0.0} ("線段2端點"), Variant=w706) -> (data=w721:T26)  [unwired: 1 in, 1 out]
        n270 = Variant To Data(type=T29 {"左X分量"=0.0, "左Y分量"=0.0, "右X分量"=0.0, "右Y分量"=0.0, "pixel轉mm(左)"=0.0, "offect總值 out"={"總值左out"=0.0, "總值右out "=0.0}} ("output cluster"), Variant=w717) -> (data=w719:T29)  [unwired: 1 in, 1 out]
        n271 = Variant To Data(type=T28 {{"掃描速度"=0, "功率"=0, "切割刀數"=0, "角度"=0.0}, {"掃描速度2"=0, "功率2"=0, "切割刀數2"=0, "角度2"=0.0}, {"掃描速度3"=0, "功率3"=0, "切割刀數3"=0, "角度3"=0.0}, {"掃描速度4"=0, "功率4"=0, "切割刀數4"=0, "角度4"=0.0}, {"掃描速度5"=0, "功率5"=0, "切割刀數5"=0}} ("output cluster"), Variant=w691) -> (data=w690:T28)  [unwired: 1 in, 1 out]
        n272 = Unbundle By Name(w719) -> ("pixel轉mm(左)"=w722:dbl)
        n273 = Unbundle(w690) -> (w688:T37, w687:T38)  [unwired: 3 out]
        n274 = call "量測_VI_邊長度.vi"("pixel 轉 mm"=w722, "右邊值"=w721, "左邊值"=w720) -> ("右邊長度"=w701:dbl, "左邊長度"=w704:dbl)  [unwired: 7 in]
        n275 = Unbundle(w688) -> ("掃描速度"=w702:i32, "功率"=w703:i32, "切割刀數"=w698:i32, "角度"=w697:dbl)
        n276 = Unbundle(w687) -> ("掃描速度2"=w699:i32, "功率2"=w700:i32, "角度2"=w696:dbl)  [unwired: 1 out]
        n277 = stacked-sequence {
          seq-local: [w739 _ _ _ _ _ _] -> [_ w745 _ _ _ _ _]
          seq-local: [_ w745 _ _ _ _ _] -> [_ _ w757 _ _ _ _]
          seq-local: [_ _ w755 _ _ _ _] -> [_ _ _ w761 _ _ _]
          seq-local: [_ _ _ w761 _ _ _] -> [_ _ _ _ w765 _ _]
          seq-local: [_ _ _ _ w764 _ _] -> [_ _ _ _ _ w773 _]
          seq-local: [_ _ _ _ w763 _ _] -> [_ _ _ _ _ w772 _]
          seq-local: [_ _ _ _ _ w773 _] -> [_ _ _ _ _ _ w777]
          seq-local: [_ _ _ _ _ w772 _] -> [_ _ _ _ _ _ w776]
          tunnel: w686 -> [w738 _ _ _ _ _ _]
          tunnel: w683 -> [w734 _ _ _ _ _ _]
          tunnel: w685 -> [_ _ w754 _ _ _ _]
          tunnel: w684 -> [_ _ w750 _ _ _ _]
          tunnel: w704 -> [w733 _ _ _ _ _ _]
          tunnel: w703 -> [w737 _ _ _ _ _ _]
          tunnel: w702 -> [w736 _ _ _ _ _ _]
          tunnel: w701 -> [_ _ w749 _ _ _ _]
          tunnel: w700 -> [_ _ w753 _ _ _ _]
          tunnel: w699 -> [_ _ w752 _ _ _ _]
          tunnel: w698 -> [_ _ _ _ _ _ w775]
          tunnel: w697 -> [w735 _ _ _ _ _ _]
          tunnel: w696 -> [_ _ w751 _ _ _ _]
          frame #0 {
            n278 = Subtract(x=w734, y=w733) -> (x-y=w732:dbl)
            n279 = Add(x=w732, y=0.9) -> (x+y=w730:dbl)
            n280 = call "RS232_命令(2條直線要寫入雷射的)_VI.vi"("量測值Array(X)"=w738, "量測值Array(Y)"=w730, "線段"=enum16{"左邊線段", "右邊線段"}."左邊線段", "功率左"=w737, "角度(左)"=w735, "掃描速率(刀速) 左"=w736, "線段長度左"=w733) -> ("命令字串"=w741:string, "error out"=w742:errorcluster)  [unwired: 11 in]
            n281 = call "雷射_FGV.vi"("Enum"=T27."寫入雷射XY座標值與角度", "error in"=w742, "命令字串"=w741) -> ("error out"=w739:errorcluster)  [unwired: 6 in, 2 out]
          }
          frame #1 {
            n282 = Wait (ms)(milliseconds to wait=u32 350) -> ()  [unwired: 1 out]
          }
          frame #2 {
            n283 = Subtract(x=w750, y=w749) -> (x-y=w748:dbl)
            n284 = Subtract(x=w748, y=0.0) -> (x-y=w746:dbl)
            n285 = call "RS232_命令(2條直線要寫入雷射的)_VI.vi"("量測值Array(X)"=w754, "量測值Array(Y)"=w746, "功率右"=w753, "掃描速率(刀速)右"=w752, "error in (no error)"=w757, "線段"=enum16{"左邊線段", "右邊線段"}."右邊線段", "角度(右)"=w751, "線段長度右"=w749) -> ("命令字串"=w759:string, "error out"=w756:errorcluster)  [unwired: 10 in]
            n286 = call "雷射_FGV.vi"("Enum"=T27."寫入雷射XY座標值與角度", "error in"=w756, "命令字串"=w759) -> ("error out"=w755:errorcluster)  [unwired: 6 in, 2 out]
          }
          frame #3 {
            n287 = Wait (ms)(milliseconds to wait=u32 350) -> ()  [unwired: 1 out]
          }
          frame #4 {
            n288 = disable-structure shown="Enabled" {
              disable-tunnel: w765 -> [w769 w771]
              disable-tunnel: [w767 w771] -> w764
              disable-tunnel: [w766 _] -> w763
              frame Disabled {
                # "讀出program值"
                n289 = call "雷射_FGV.vi"("Enum"=T27."寫入雷射XY座標值與角度", "error in"=w769, "命令字串"="F1,0000") -> ("error out"=w767:errorcluster, "回復訊息"=w766:string)  [unwired: 6 in, 1 out]
              }
              frame Enabled {
              }
            }
          }
          frame #5 {
            n290 = disable-structure shown="Disabled" {
              frame Disabled {
                n291 = Wait (ms)(milliseconds to wait=u32 350) -> ()  [unwired: 1 out]
              }
              frame Enabled {
              }
            }
          }
          frame #6 {
            n292 = disable-structure shown="Disabled" {
              disable-tunnel: w777 -> [w784 _]
              disable-tunnel: w776 -> [w783 _]
              disable-tunnel: w775 -> [w778 _]
              frame Disabled {
                # "將讀出值F1，0及刀數替換"
                n293 = call "RS232_命令(刀數).vi"("error in (no error)"=w784, "program"=enum16{"0000", "0002"}."0000", "刀數"=w778, "回復訊息 3"=w783) -> ("error out"=w781:errorcluster, "result string 3"=w779:string)  [unwired: 6 in]
                n294 = call "雷射_FGV.vi"("Enum"=T27."寫入雷射XY座標值與角度", "error in"=w781, "命令字串"=w779) -> ()  [unwired: 6 in, 3 out]
              }
              frame Enabled {
              }
            }
          }
        }
      }
      frame "      5.2雷射-寫入數值2" {
        n295 = for {
          tunnel: [w891] -> w821 mode=indexing
          tunnel: string[] ["邊L座標", "邊R座標", "量測2"] -> [w890] mode=indexing
          n296 = call "Main_FGV_Data.vi"("Action_Data"=Action_Data."Get Data", "Data name"=w890) -> ("Data  Out"=w891:cluster{"Data name":string, "Data":variant})  [unwired: 8 in, 1 out]
        }
        n297 = call "Main_FGV_Data.vi"("Action_Data"=Action_Data."Get Data", "Data name"="量測2") -> ("Data  Out"=w830:cluster{"Data name":string, "Data":variant})  [unwired: 8 in, 1 out]
        n298 = call "Main_FGV_Data.vi"("Action_Data"=Action_Data."Get Data", "Data name"="參數設定") -> ("Data  Out"=w797:cluster{"Data name":string, "Data":variant})  [unwired: 8 in, 1 out]
        n299 = Unbundle By Name(w830) -> ("Data"=w829:variant)
        n300 = Index Array(array=w821, index #1=0 ("index"), index #2=1 ("index"), index #3=2 ("index")) -> (element #1=w818:cluster{"Data name":string, "Data":variant}, element #2=w814:cluster{"Data name":string, "Data":variant}, element #3=w823:cluster{"Data name":string, "Data":variant})
        n301 = Unbundle By Name(w797) -> ("Data"=w796:variant)
        n302 = Unbundle By Name(w818) -> ("Data"=w816:variant)
        n303 = Variant To Data(type=T30 {"左X分量"=0.0, "左Y分量"=0.0, "右X分量"=0.0, "右Y分量"=0.0, "pixel轉mm(右)"=0.0, "offect總值 out"={"總值左out"=0.0, "總值右out "=0.0}} ("output cluster"), Variant=w829) -> (data=w828:T30)  [unwired: 1 in, 1 out]
        n304 = Unbundle By Name(w814) -> ("Data"=w813:variant)
        n305 = Unbundle By Name(w823) -> ("Data"=w824:variant)
        n306 = Variant To Data(type=T26 {"點1 (Pixels)"={"X"=0.0, "Y"=0.0}, "點2 (Pixels)"={"X"=0.0, "Y"=0.0}, "Angle (Pixel)"=0.0} ("線段2端點"), Variant=w816) -> (data=w826:T26)  [unwired: 1 in, 1 out]
        n307 = Variant To Data(type=T26 {"點1 (Pixels)"={"X"=0.0, "Y"=0.0}, "點2 (Pixels)"={"X"=0.0, "Y"=0.0}, "Angle (Pixel)"=0.0} ("線段2端點"), Variant=w813) -> (data=w827:T26)  [unwired: 1 in, 1 out]
        n308 = Variant To Data(type=T30 {"左X分量"=0.0, "左Y分量"=0.0, "右X分量"=0.0, "右Y分量"=0.0, "pixel轉mm(右)"=0.0, "offect總值 out"={"總值左out"=0.0, "總值右out "=0.0}} ("output cluster"), Variant=w824) -> (data=w825:T30)  [unwired: 1 in, 1 out]
        n309 = Unbundle By Name(w828) -> ("左X分量"=w790:dbl, "左Y分量"=w788:dbl, "右X分量"=w791:dbl, "右Y分量"=w789:dbl)
        n310 = Unbundle By Name(w825) -> ("pixel轉mm(右)"=w810:dbl)
        n311 = Variant To Data(type=T28 {{"掃描速度"=0, "功率"=0, "切割刀數"=0, "角度"=0.0}, {"掃描速度2"=0, "功率2"=0, "切割刀數2"=0, "角度2"=0.0}, {"掃描速度3"=0, "功率3"=0, "切割刀數3"=0, "角度3"=0.0}, {"掃描速度4"=0, "功率4"=0, "切割刀數4"=0, "角度4"=0.0}, {"掃描速度5"=0, "功率5"=0, "切割刀數5"=0}} ("output cluster"), Variant=w796) -> (data=w795:T28)  [unwired: 1 in, 1 out]
        n312 = call "量測_VI_邊長度.vi"("pixel 轉 mm"=w810, "右邊值"=w827, "左邊值"=w826) -> ("右邊長度"=w805:dbl, "左邊長度"=w809:dbl)  [unwired: 7 in]
        n313 = Unbundle(w795) -> (w793:T39, w792:T40)  [unwired: 3 out]
        n314 = Unbundle(w793) -> ("掃描速度3"=w808:i32, "功率3"=w807:i32, "切割刀數3"=w801:i32, "角度3"=w806:dbl)
        n315 = Unbundle(w792) -> ("掃描速度4"=w803:i32, "功率4"=w802:i32, "角度4"=w804:dbl)  [unwired: 1 out]
        n316 = stacked-sequence {
          seq-local: [w844 _ _ _ _ _ _] -> [_ w850 _ _ _ _ _]
          seq-local: [_ w850 _ _ _ _ _] -> [_ _ w862 _ _ _ _]
          seq-local: [_ _ w860 _ _ _ _] -> [_ _ _ w866 _ _ _]
          seq-local: [_ _ _ w866 _ _ _] -> [_ _ _ _ w870 _ _]
          seq-local: [_ _ _ _ w869 _ _] -> [_ _ _ _ _ w878 _]
          seq-local: [_ _ _ _ w868 _ _] -> [_ _ _ _ _ w877 _]
          seq-local: [_ _ _ _ _ w878 _] -> [_ _ _ _ _ _ w882]
          seq-local: [_ _ _ _ _ w877 _] -> [_ _ _ _ _ _ w881]
          tunnel: w791 -> [w843 _ _ _ _ _ _]
          tunnel: w789 -> [w839 _ _ _ _ _ _]
          tunnel: w790 -> [_ _ w859 _ _ _ _]
          tunnel: w788 -> [_ _ w855 _ _ _ _]
          tunnel: w809 -> [w838 _ _ _ _ _ _]
          tunnel: w808 -> [w842 _ _ _ _ _ _]
          tunnel: w807 -> [w841 _ _ _ _ _ _]
          tunnel: w806 -> [w840 _ _ _ _ _ _]
          tunnel: w805 -> [_ _ w854 _ _ _ _]
          tunnel: w804 -> [_ _ w858 _ _ _ _]
          tunnel: w803 -> [_ _ w857 _ _ _ _]
          tunnel: w802 -> [_ _ w856 _ _ _ _]
          tunnel: w801 -> [_ _ _ _ _ _ w880]
          frame #0 {
            n317 = Subtract(x=w839, y=w838) -> (x-y=w835:dbl)
            n318 = Add(x=w835, y=1.5) -> (x+y=w837:dbl)
            n319 = call "RS232_命令(2條直線要寫入雷射的)_VI.vi"("量測值Array(X)"=w843, "量測值Array(Y)"=w837, "線段"=enum16{"左邊線段", "右邊線段"}."左邊線段", "功率左"=w841, "角度(左)"=w840, "掃描速率(刀速) 左"=w842, "線段長度左"=w838) -> ("命令字串"=w846:string, "error out"=w847:errorcluster)  [unwired: 11 in]
            n320 = call "雷射_FGV.vi"("Enum"=T27."寫入雷射XY座標值與角度", "error in"=w847, "命令字串"=w846) -> ("error out"=w844:errorcluster)  [unwired: 6 in, 2 out]
          }
          frame #1 {
            n321 = Wait (ms)(milliseconds to wait=u32 350) -> ()  [unwired: 1 out]
          }
          frame #2 {
            n322 = Subtract(x=w855, y=w854) -> (x-y=w853:dbl)
            n323 = Subtract(x=w853, y=0.5) -> (x-y=w851:dbl)
            n324 = call "RS232_命令(2條直線要寫入雷射的)_VI.vi"("量測值Array(X)"=w859, "量測值Array(Y)"=w851, "功率右"=w856, "掃描速率(刀速)右"=w857, "error in (no error)"=w862, "線段"=enum16{"左邊線段", "右邊線段"}."右邊線段", "角度(右)"=w858, "線段長度右"=w854) -> ("命令字串"=w864:string, "error out"=w861:errorcluster)  [unwired: 10 in]
            n325 = call "雷射_FGV.vi"("Enum"=T27."寫入雷射XY座標值與角度", "error in"=w861, "命令字串"=w864) -> ("error out"=w860:errorcluster)  [unwired: 6 in, 2 out]
          }
          frame #3 {
            n326 = Wait (ms)(milliseconds to wait=u32 350) -> ()  [unwired: 1 out]
          }
          frame #4 {
            n327 = disable-structure shown="Enabled" {
              disable-tunnel: w870 -> [w874 w876]
              disable-tunnel: [w872 w876] -> w869
              disable-tunnel: [w871 _] -> w868
              frame Disabled {
                # "讀出program值"
                n328 = call "雷射_FGV.vi"("Enum"=T27."寫入雷射XY座標值與角度", "error in"=w874, "命令字串"="F1,0000") -> ("error out"=w872:errorcluster, "回復訊息"=w871:string)  [unwired: 6 in, 1 out]
              }
              frame Enabled {
              }
            }
          }
          frame #5 {
            n329 = disable-structure shown="Disabled" {
              frame Disabled {
                n330 = Wait (ms)(milliseconds to wait=u32 350) -> ()  [unwired: 1 out]
              }
              frame Enabled {
              }
            }
          }
          frame #6 {
            n331 = disable-structure shown="Disabled" {
              disable-tunnel: w882 -> [w889 _]
              disable-tunnel: w881 -> [w888 _]
              disable-tunnel: w880 -> [w883 _]
              frame Disabled {
                # "將讀出值F1，0及刀數替換"
                n332 = call "RS232_命令(刀數).vi"("error in (no error)"=w889, "program"=enum16{"0000", "0002"}."0000", "刀數"=w883, "回復訊息 3"=w888) -> ("error out"=w886:errorcluster, "result string 3"=w884:string)  [unwired: 6 in]
                n333 = call "雷射_FGV.vi"("Enum"=T27."寫入雷射XY座標值與角度", "error in"=w886, "命令字串"=w884) -> ()  [unwired: 6 in, 3 out]
              }
              frame Enabled {
              }
            }
          }
        }
      }
      frame "      5.3雷射-寫入刀數" {
        n334 = call "Main_FGV_Data.vi"("Action_Data"=Action_Data."Get Data", "Data name"="參數設定") -> ("Data  Out"=w898:cluster{"Data name":string, "Data":variant})  [unwired: 8 in, 1 out]
        n335 = Unbundle By Name(w898) -> ("Data"=w897:variant)
        n336 = flat-sequence {
          tunnel: [w909] -> w903
          tunnel: [w908] -> w902
          tunnel: [w913] -> w904
          tunnel: w903 -> [w913]
          tunnel: w902 -> [w912]
          tunnel: [w912] -> w901
          tunnel: w904 -> [w918]
          tunnel: w901 -> [w916]
          tunnel: w900 -> [w915]
          frame #0 {
            n337 = Wait (ms)(milliseconds to wait=u32 350) -> ()  [unwired: 1 out]
          }
          frame #1 {
            # "讀出program值"
            n338 = call "雷射_FGV.vi"("Enum"=T27."寫入雷射XY座標值與角度", "命令字串"="F1,0000") -> ("error out"=w909:errorcluster, "回復訊息"=w908:string)  [unwired: 7 in, 1 out]
          }
          frame #2 {
            n339 = Wait (ms)(milliseconds to wait=u32 350) -> ()  [unwired: 1 out]
          }
          frame #3 {
            # "將讀出值F1，0及刀數替換"
            n340 = call "RS232_命令(刀數).vi"("error in (no error)"=w918, "program"=enum16{"0000", "0002"}."0000", "刀數"=w915, "回復訊息 3"=w916) -> ("error out"=w917:errorcluster, "result string 3"=w920:string)  [unwired: 6 in]
            n341 = call "雷射_FGV.vi"("Enum"=T27."寫入雷射XY座標值與角度", "error in"=w917, "命令字串"=w920) -> ()  [unwired: 6 in, 3 out]
          }
        }
        n342 = Variant To Data(type=T31 {{"掃描速度"=0, "功率"=0, "切割刀數"=0, "角度"=0.0}, {"掃描速度2"=0, "功率2"=0, "切割刀數"=0, "角度2"=0.0}, {"掃描速度3"=0, "功率3"=0, "切割刀數3"=0, "角度3"=0.0}, {"掃描速度4"=0, "功率4"=0, "切割刀數3"=0, "角度4"=0.0}, {"掃描速率(刀速) "=0, "功率"=0, "刀數"=0}} ("output cluster"), Variant=w897) -> (data=w896:T31)  [unwired: 1 in, 1 out]
        n343 = Unbundle(w896) -> (w895:T37)  [unwired: 4 out]
        n344 = Unbundle(w895) -> ("切割刀數"=w900:i32)  [unwired: 3 out]
      }
      frame "      5.4雷射-讀出數值" {
      }
      frame "      5.5雷射-切換" {
        n345 = flat-sequence {
          frame #0 {
            n346 = Wait (ms)(milliseconds to wait=u32 350) -> ()  [unwired: 1 out]
          }
          frame #1 {
            n347 = call "雷射_FGV.vi"("Enum"=T27."運行切換", "PROGRAM"=enum16{"0000", "0002"}."0000") -> ()  [unwired: 7 in, 3 out]
          }
        }
      }
      frame "      5.6雷射-雷射觸發" {
        n348 = flat-sequence {
          tunnel: [w935] -> w929
          tunnel: w929 -> [_]
          frame #0 {
            n349 = Wait (ms)(milliseconds to wait=u32 350) -> ()  [unwired: 1 out]
          }
          frame #1 {
            n350 = call "雷射_FGV.vi"("Enum"=T27."雷射準備訊號") -> ("error out"=w936:errorcluster)  [unwired: 8 in, 2 out]
            n351 = call "雷射_FGV.vi"("Enum"=T27."雷射觸發", "error in"=w936) -> ("error out"=w935:errorcluster)  [unwired: 7 in, 2 out]
          }
          frame #2 {
            n352 = Wait (ms)(milliseconds to wait=u32 500) -> ()  [unwired: 1 out]
          }
        }
        n353 = disable-structure shown="Disabled" {
          frame Disabled {
            n354 = flat-sequence {
              tunnel: [w940] -> w938
              tunnel: w938 -> [_]
              frame #0 {
                n355 = Wait (ms)(milliseconds to wait=u32 350) -> ()  [unwired: 1 out]
              }
              frame #1 {
                n356 = call "雷射_FGV.vi"("Enum"=T32."雷射準備訊號") -> ("error out"=w941:errorcluster)  [unwired: 8 in, 2 out]
                n357 = call "雷射_FGV.vi"("Enum"=T32."雷射觸發", "error in"=w941) -> ("error out"=w940:errorcluster)  [unwired: 7 in, 2 out]
              }
              frame #2 {
                n358 = Wait (ms)(milliseconds to wait=u32 850) -> ()  [unwired: 1 out]
              }
            }
          }
          frame Enabled {
          }
        }
      }
      frame "      5.7雷射-關閉" {
        n359 = call "雷射_FGV.vi"("Enum"=T27."RS232_Close") -> ()  [unwired: 8 in, 3 out]
      }
      frame "6.0功能-檔案" {
      }
      frame "       6.1檔案-初始化" {
        n360 = call "Main_FGV_Data.vi"("Action_Data"=Action_Data."Initialize") -> ()  [unwired: 9 in, 2 out]
      }
      frame "       6.2檔案-儲存檔案" {
        (unwired) path "C:/Users/jyun.huang.MINAIK/Desktop/四穴雷切/連線測試(量測)/Untitled 2 2013/Measure/Data(近點)/Data(近點)" ("file (use dialog)")
        n361 = for {
          tunnel: [w959] -> w954 mode=indexing
          tunnel: string[] ["量測1", "量測2"] -> [w958] mode=indexing
          n362 = call "Main_FGV_Data.vi"("Action_Data"=Action_Data."Get Data", "Data name"=w958) -> ("Data  Out"=w959:cluster{"Data name":string, "Data":variant})  [unwired: 8 in, 1 out]
        }
        n363 = Write to Binary File(file (use dialog)=path "C:/Users/noname/Desktop/Main-Page/四穴雷切/Data資料夾/量測進點 Data/Data(近點)", data=w954) -> ()  [unwired: 4 in, 3 out]
      }
      frame "       6.3檔案-開啟檔案(setting)" {
        (unwired) path "C:/Users/jyun.huang.MINAIK/Desktop/四穴雷切/Setting/Data/TresselData" ("setting 路徑")
        w961 = path "C:/Users/noname/Desktop/Main-Page/四穴雷切/Data資料夾/setting Data/TresselData" ("setting 路徑")
        n364 = call "Image FGV.vi"("Image action"=Image_action."讀取圖片", "圖片名稱"="Pattern_L") -> ("Image Out"=w977:T3)  [unwired: 8 in, 1 out]
        n365 = call "Image FGV.vi"("Image action"=Image_action."讀取圖片", "圖片名稱"="Pattern_R") -> ("Image Out"=w975:T3)  [unwired: 8 in, 1 out]
        n366 = call "Main_FGV_Data.vi"("Action_Data"=Action_Data."Initialize") -> ("Data Array out"=w984:cluster{"Data name":string, "Data":variant}[])  [unwired: 9 in, 1 out]
        n367 = Strip Path(path=w961) -> (stripped path=w968:path, name=w969:string)
        n368 = Strip Path(path=w961) -> (stripped path=w967:path, name=w966:string)
        n369 = Read from Binary File(5:w984, 11:w961) -> (0:w962:errorcluster, 2:w979:cluster{"Data name":string, "Data":variant}[])  [unwired: 4 in, 2 out]
        n370 = Concatenate Strings(w969, "-" ("string"), "Pattern_L.png" ("name or relative path")) -> (w971:string)
        n371 = Concatenate Strings(w966, "-" ("string"), "Pattern_R.png" ("name or relative path")) -> (w970:string)
        n372 = Build Path(base path=w968, name or relative path=w971) -> (appended path=w978:path)
        n373 = Build Path(base path=w967, name or relative path=w970) -> (appended path=w976:path)
        n374 = for {
          tunnel: w979 -> [w993] mode=indexing
          n375 = Unbundle(w993) -> ("Data name"=w991:string)  [unwired: 1 out]
          n376 = call "Main_FGV_Data.vi"("Action_Data"=Action_Data."Set Data", "Data In"=w993, "Data name"=w991) -> ()  [unwired: 7 in, 2 out]
        }
        n377 = call "IMAQ Read Image And Vision Info"("File Path"=w978, "Image"=w977) -> ("error out"=w963:errorcluster)  [unwired: 7 in, 2 out]
        n378 = call "IMAQ Read Image And Vision Info"("File Path"=w976, "Image"=w975) -> ("error out"=w964:errorcluster)  [unwired: 7 in, 2 out]
        n379 = Enqueue Element(queue=w990, element=連線測試_Control_Main_Action."       3.2影像-更新影像", error in (no error)=w989) -> (queue out=w988:refnum<queue>, error out=w987:errorcluster)  [unwired: 1 in, 1 out]
      }
      frame "       6.3檔案-開啟檔案(點檢)" {
        w994 = path "C:/Users/noname/Desktop/Main-Page/四穴雷切/Data資料夾/點檢Data" ("點檢路徑")
        n380 = call "Main_FGV_Data.vi"("Action_Data"=Action_Data."Idle") -> ("Data Array out"=w999:cluster{"Data name":string, "Data":variant}[])  [unwired: 9 in, 1 out]
        n381 = call "Main_FGV_Data.vi"("Action_Data"=Action_Data."Idle") -> ("Data Array out"=w1004:cluster{"Data name":string, "Data":variant}[])  [unwired: 9 in, 1 out]
        n382 = Build Path(base path=w994, name or relative path="點檢Data右") -> (appended path=w1000:path)
        n383 = Build Path(base path=w994, name or relative path="點檢Data左") -> (appended path=w1003:path)
        n384 = Read from Binary File(5:w1004, 11:w1003) -> (0:w1006:errorcluster, 2:w1007:cluster{"Data name":string, "Data":variant}[])  [unwired: 4 in, 2 out]
        n385 = for {
          tunnel: w1007 -> [w1014] mode=indexing
          tunnel: w1006 -> [w1013]
          tunnel: [w1013] -> w995
          n386 = Unbundle(w1014) -> ("Data name"=w1015:string)  [unwired: 1 out]
          n387 = call "Main_FGV_Data.vi"("Action_Data"=Action_Data."Set Data", "Data In"=w1014, "Data name"=w1015) -> ()  [unwired: 7 in, 2 out]
        }
        n388 = Read from Binary File(5:w999, 8:w995, 11:w1000) -> (0:w997:errorcluster, 2:w996:cluster{"Data name":string, "Data":variant}[])  [unwired: 3 in, 2 out]
        n389 = for {
          tunnel: w996 -> [w1010] mode=indexing
          tunnel: w997 -> [_]
          n390 = Unbundle(w1010) -> ("Data name"=w1011:string)  [unwired: 1 out]
          n391 = call "Main_FGV_Data.vi"("Action_Data"=Action_Data."Set Data", "Data In"=w1010, "Data name"=w1011) -> ()  [unwired: 7 in, 2 out]
        }
      }
      frame "       6.3檔案-開啟檔案(近點)" {
        n392 = call "Main_FGV_Data.vi"("Action_Data"=Action_Data."Idle") -> ("Data Array out"=w1019:cluster{"Data name":string, "Data":variant}[])  [unwired: 9 in, 1 out]
        n393 = Read from Binary File(5:w1019, 11:path "C:/Users/noname/Desktop/Main-Page/四穴雷切/Data資料夾/量測進點 Data/Data(近點)" ("量測路徑")) -> (2:w1017:cluster{"Data name":string, "Data":variant}[])  [unwired: 4 in, 3 out]
        n394 = for {
          tunnel: w1017 -> [w1023] mode=indexing
          n395 = Unbundle(w1023) -> ("Data name"=w1024:string)  [unwired: 1 out]
          n396 = call "Main_FGV_Data.vi"("Action_Data"=Action_Data."Set Data", "Data In"=w1023, "Data name"=w1024) -> ()  [unwired: 7 in, 2 out]
        }
      }
      frame "       6.4檔案-匯入檔案(近點)" {
        n397 = call "Main_FGV_Data.vi"("Action_Data"=Action_Data."Get Data", "Data name"="量測1") -> ("Data  Out"=w1046:cluster{"Data name":string, "Data":variant})  [unwired: 8 in, 1 out]
        n398 = call "Main_FGV_Data.vi"("Action_Data"=Action_Data."Get Data", "Data name"="量測2") -> ("Data  Out"=w1042:cluster{"Data name":string, "Data":variant})  [unwired: 8 in, 1 out]
        n399 = Unbundle By Name(w1046) -> ("Data"=w1047:variant)
        n400 = Unbundle By Name(w1042) -> ("Data"=w1043:variant)
        n401 = Variant To Data(type=T34 {"Distances左水平(mm)"=0.0, "Distance左垂直(mm)"=0.0, "Distances右水平(mm)"=0.0, "Distance右垂直(mm)"=0.0, "pixel轉mm(左)"=0.0, "總值 out"={"總值左out"=0.0, "總值右out "=0.0}} ("output cluster"), Variant=w1047) -> (data=w1035:T34, error out=w1039:errorcluster)  [unwired: 1 in]
        n402 = Variant To Data(error in=w1039, type=T33 {"Distances左水平(mm)"=0.0, "Distance左垂直(mm)"=0.0, "Distances右水平(mm)"=0.0, "Distance右垂直(mm)"=0.0, "pixel轉mm(右)"=0.0, "總值 out"={"總值左out"=0.0, "總值右out "=0.0}} ("output cluster 2"), Variant=w1043) -> (data=w1034:T33, error out=w1038:errorcluster)
        n403 = Unbundle By Name(w1034) -> ("pixel轉mm(右)"=w1029:dbl, "總值 out"=w1028:cluster{"總值左out":dbl, "總值右out ":dbl})
        n404 = Unbundle By Name(w1035) -> ("pixel轉mm(左)"=w1033:dbl, "總值 out"=w1032:cluster{"總值左out":dbl, "總值右out ":dbl})
        n405 = Unbundle(w1028) -> ("總值左out"=w1027:dbl, "總值右out"=w1026:dbl)
        n406 = Unbundle(w1032) -> ("總值左out"=w1031:dbl, "總值右out"=w1030:dbl)
        n407 = local write "pixel轉mm(右)"(w1029) -> ()
        n408 = local write "pixel轉mm(左)"(w1033) -> ()
        n409 = local write "總值左out 2"(w1027) -> ()
        n410 = local write "總值右out 2"(w1026) -> ()
        n411 = local write "總值右out"(w1030) -> ()
        n412 = local write "總值左out"(w1031) -> ()
      }
      frame "       6.4檔案-開啟檔案(雷射)" {
        n413 = call "Main_FGV_Data.vi"("Action_Data"=Action_Data."Idle") -> ("Data Array out"=w1051:cluster{"Data name":string, "Data":variant}[])  [unwired: 9 in, 1 out]
        n414 = Read from Binary File(5:w1051, 11:path "C:/Users/noname/Desktop/Main-Page/四穴雷切/Data資料夾/參數設定Data/參數設定" ("file (use dialog)")) -> (2:w1050:cluster{"Data name":string, "Data":variant}[])  [unwired: 4 in, 3 out]
        n415 = for {
          tunnel: w1050 -> [w1056] mode=indexing
          n416 = Unbundle(w1056) -> ("Data name"=w1057:string)  [unwired: 1 out]
          n417 = call "Main_FGV_Data.vi"("Action_Data"=Action_Data."Set Data", "Data In"=w1056, "Data name"=w1057) -> ()  [unwired: 7 in, 2 out]
        }
      }
      frame "7.0 錯誤" {
      }
      frame "8.0等待" {
      }
      frame "       8.1等待(計算時間)" {
      }
      frame "9.0離開" {
        n418 = Flush Queue(queue=w1068, error in (no error)=w1067) -> (queue out=w1065:refnum<queue>, error out=w1066:errorcluster)  [unwired: 1 out]
      }
      frame "10.0功能-機台驗證" {
      }
      frame "      10.1機台驗證-初始化" {
      }
      frame "      10.2機台驗證-檢測" {
      }
      frame "11.0對話視窗" {
      }
    }
  }
  n419 = property on="Image 2" class="ImageControl"("Image Area Size"=cluster{"Width":u32, "Height":u32} {"Width"=935, "Height"=545} ("Image Area:Size:All Elements")) -> ()  [unwired: 2 in, 2 out]
  n420 = property on="Image1" class="ImageControl"("Image Area Size"=cluster{"Width":u32, "Height":u32} {"Width"=935, "Height"=545} ("Image Area:Size:All Elements")) -> ()  [unwired: 2 in, 2 out]
  n421 = Release Queue(queue=w17, error in (no error)=w16) -> ()  [unwired: 1 in, 3 out]
